vi "RDS Shore Remote.vi"() -> ()   [LabVIEW 2015]
uses:
  Libraries/3rd Party/NMEA_GPS/NMEA_GPRMC-data.ctl
  Libraries/3rd Party/NMEA_GPS/NMEA_LatitudeDirection.ctl
  Libraries/3rd Party/NMEA_GPS/NMEA_LongitudeDirection.ctl
  Libraries/RDS Instruments/Compass/Compass Data.ctl
  Libraries/RDS Child Messages/MCB/MCB Motor Status.ctl
  Libraries/RDS Child Messages/Mission Messages/Mission Controller State Control.ctl
  RDS Mission Controller Actor/Mission Controller Navigation State.ctl
  RDS Mission Controller Actor/MissionOp.ctl
  Libraries/RDS Child Messages/Helm/Helm Status Message/Helm Status Control.ctl
  Actors/RDS Helm Actor/RDS Helm Actor/Helm State.ctl
  Libraries/RDS Child Messages/Helm/Heading Command/Heading Command Cntrl.ctl
  Libraries/RDS Child Messages/Helm/Steering Command/Steering Command Cntrl.ctl
  Libraries/RDS Child Messages/PID Gains/PID Gains Control.ctl
  Libraries/RDS Instruments/AIP/AIP Status.ctl
  Libraries/RDS Instruments/AIP/AIP States.ctl
  Libraries/RDS Instruments/Battery/Battery Data.ctl
  Libraries/RDS Child Messages/Battery Data/Battery Status.ctl
  Actors/RDS Controller Actor/RDS Controller Actor/Controller.ctl
  SR_Overview.ctl
  SR_Thermal.ctl
  RDS Mission Controller Actor/Mission Controller Settings.ctl
  Libraries/GUI/Throttles.ctl
  RDS State Tracker/RDS State/RDS State.lvclass
  Libraries/RDS Framework/RDS Message Class/RDS Message.lvclass
  Libraries/RDS Serial Handler/RDS Serial Instrument.lvclass
  RDS Q Message.ctl
  SR-J-State.ctl
  Libraries/RDS Serial Handler/RDS Serial Frame.lvclass/RDS Serial Frame.ctl
  Libraries/RDS Serial Handler/RDS Serial Instrument.lvclass/RDS Serial Instrument.ctl
  RDS State Tracker/RDS State/RDS State.lvclass/RDS State.ctl
  Libraries/RDS Framework/RDS Message Class/RDS Message.lvclass/RDS Message.ctl
  Libraries/RDS Child Messages/Controller Message/Controller Message.lvclass
  Libraries/RDS Child Messages/Controller Message/Controller Message.lvclass/Controller Message.ctl
  Libraries/RDS Child Messages/State Sample Message/State Sample Message.lvclass
  Libraries/RDS Child Messages/State Sample Message/State Sample Message.lvclass/State Sample Message.ctl
  Libraries/RDS Framework/RDS Message ID.ctl
  Libraries/RDS Child Messages/PID Gains/PID Gains Set Message.lvclass
  Libraries/RDS Child Messages/PID Gains/PID Gains Set Message.lvclass/PID Gains Set Message.ctl
  Libraries/RDS Child Messages/Helm/Steering Command/Steering Command.lvclass
  Libraries/RDS Child Messages/Helm/Steering Command/Steering Command.lvclass/Steering Command.ctl
  Libraries/RDS Child Messages/Controller Message/Controller Message Type.ctl
  Libraries/RDS Child Messages/AIP Set Min Depth Message/AIP Set Min Depth Message.lvclass
  Libraries/RDS Child Messages/AIP Set Min Depth Message/AIP Set Min Depth Message.lvclass/AIP Set Min Depth Message.ctl
  Libraries/RDS Child Messages/Helm/Helm Limiter Message/Helm Limiter Msg.lvclass
  Libraries/RDS Child Messages/Helm/Helm Limiter Message/Helm Limiter Msg.lvclass/Helm Limiter Msg.ctl
  Libraries/RDS Framework/RDS Message Class/AIP Command.lvclass
  Libraries/RDS Framework/RDS Message Class/AIP Command Control.ctl
  Libraries/RDS Framework/RDS Message Class/AIP Command.lvclass/AIP Command.ctl
  <vilib>/Utility/inputDevices.llb/closeJoystick.vi
  Libraries/RDS Serial Handler/RDS Serial Frame.lvclass
  LSR Instrument Actor/LSR Instrument/LSR Instrument.lvlib
  LSR Transmission/LSR Transmission.lvlib
  Shore Library.lvlib
  Libraries/RDS Child Messages/RDS Child Messages.lvlib
  Compass Instrument/Compass Instrument.lvlib
  RDS Mission Controller Actor/RDS Mission Controller Actor.lvlib
  Actors/RDS Controller Actor/RDS Controller Actor/RDS Controller Actor.lvlib
  Libraries/RDS Instruments/RDS Instrument Library.lvlib
  Actors/RDS Helm Actor/RDS Helm Actor.lvlib
  Libraries/3rd Party/NMEA_GPS/NMEA.lvlib
  Libraries/RDS Child Messages/Mission Messages/Mission Controller State Message.lvclass
  Libraries/Geo/RDS Libraries.lvlib
panel:
  in  "Track":cluster{"Long":dbl[], "Lat":dbl[]}
  in  "btn_mission_maker":bool
  out "Joystick Connected":bool
  out "iHasControl":bool
  out "AIP controls":T1
  out "Seconds Ago":dbl format="%#.0g"
  out "Last Status Message":timestamp
  out "RoboDolf State":T2
  in  "Connect Joystick":bool
  out "LSR Connected":bool
  in  "Digi Connect":bool
  in  "Digi Serial Port":refnum<visa-resource-name>="COM11"
  in  "Tab Control":T3(tab)
  out "Overview":T4 {"Distance to Target" format="%.01f [meters]"; "Longitude" format="%.6g"; "Latitude" format="%.6g"; "Water Temp" format="%.0f [celcius]"; "Pitch" scale=45.0..-45.0; "Roll" scale=-20.0..20.0; "Current" format="%02.2f [amps]"; "Voltage" format="%02.2f [volts]"; "Capacity" format="%_1f [Percent]"; "Water Depth" format="%.01f [meters]"; "GPS Speed" format="%.01f [knots]"; "Compass" scale=0.36..360.0}
  out "Tx packet  length":i32(graph)
  out "Compass Data":T5
  out "GPRMC-data":T6={"TimeStamp"=timestamp(0 s since 1904-01-01), "Validity"=FALSE, "Latitude"=0.0, "Latitude-Direction"=enum."North", "Longitude"=0.0, "Longitude-Direction"=enum."East", "Speed in knots"=0.0, "True course"=0.0, "Date Stamp"=timestamp(0 s since 1904-01-01), "Magnetic Variation (East/West)"=0.0, "GPS Latitude"=0.0, "GPS Longitude"=0.0} {"GPS Longitude" format="%.6f"; "GPS Latitude" format="%.6f"; "Magnetic Variation (East/West)" format="%.02f [deg]"; "Date Stamp" format="%<%x>T"; "True course" format="%.02f [deg]"; "Speed in knots" format="%.02f [kts]"; "Longitude" format="%0.4f [long]"; "Latitude" format="%.04f [lat]"; "TimeStamp" format="%<%.2X>T"}
  in  "Compass Mag Dev":dbl
  in  "btn_set_mag_dev":bool
  in  "AIP Stop":bool
  in  "AIP Stow":bool
  in  "AIP Deploy":bool
  out "AS":bool
  out "FS":bool
  out "AP":bool
  out "FP":bool
  out "AIP Status":T9
  in  "AIP JD FP":bool
  in  "AIP JS FP":bool
  in  "AIP JS FS":bool
  in  "AIP JD FS":bool
  in  "AIP JD AP":bool
  in  "AIP JD AS":bool
  in  "AIP JS AS":bool
  in  "AIP JS AP":bool
  in  "AIP D FP":bool
  in  "AIP D FP 4":bool
  in  "AIP D AP":bool
  in  "AIP D FS":bool
  in  "AIP S AS":bool
  in  "AIP S AP":bool
  in  "AIP S FP":bool
  in  "AIP S FS":bool
  in  "AIP Min Depth":dbl
  in  "btn_set_aip_min_depth":bool
  out "Throttles":T11 {"STBD" scale=-1000.0..1000.0; "Port" scale=-1000.0..1000.0}
  out "Rudder Chart":sgl(graph)
  out "Hdng Chart":cluster{"Heading":sgl, "Current Heading":dbl}(graph) caption="Desired and Actual Heading Chart"
  out "Helm Status":T12 {"Gains"."D (Td)" format="%#_9f"; "Gains"."I (Ti)" format="%#_9f"; "Gains"."P (Kc)" format="%#.9f"}
  in  "btn_limiter_set":bool
  in  "Limter":dbl(slide) min=0.0 max=100.0 scale=0.0..100.0
  in  "Gains":T16 {"D (Td)" format="%#_9f"; "I (Ti)" format="%#_9f"; "P (Kc)" format="%#.9f"}
  in  "btn_gains set":bool
  in  "Steering Command":T15
  in  "btn_Send-Steer":bool
  in  "btn_show_annotes":bool caption="Show Annotes"
  in  "btn_show_loaded":bool caption="Show Loaded"
  in  "btn_upload_mission":bool
  in  "btn_show_buffer_1":bool caption="Show"
  in  "btn_load_buff_mission":bool
  out "XY Graph":cluster{dbl[], dbl[]}[](graph)
  out "Mission Controller State":T17 {"Mission"."GPS Longitude" format="%.6g"; "Mission"."GPS Latitude" format="%.6g"}
  in  "btn_mission_ReqControl":bool
  in  "btn_send settings":bool
  in  "Mission Controller Settings":T20
  in  "btn_mission_Relinquish":bool
  in  "btn_set_op_run":bool
  in  "MissionOp Index":i32
  in  "btn_Turneffe":bool
  in  "btn_beach1":bool
  in  "btn_beach 2":bool
  in  "btn_save_track":bool
  out "Mission Buffer":T19[](array[typedef]) {"GPS Longitude" format="%.6g"; "GPS Latitude" format="%.6g"}
  out "Voltage Chart":T21(graph)
  out "Pow Cap Chart":cluster{"Pack Current":sgl, "Pack Capacity":sgl}(graph) caption="Power and Capacity Chart"
  out "Battery Pack Info":T22
  out "Port Motor Data":T24
  out "STBD Motor":T24
  out "Thermal":T25
  out "Thermal WF":sgl[](graph)
  in  "btn-emergency-shutdown":bool
  in  "Shutdown Safety":bool
  in  "stop":bool
  # "SAMMUT TECHNOLOGIES LLC"
  # "RoboDolf State"
  # "Batteries"
  # "Actual Heading"
  # "Desired Heading"
  # "Throttle"
  # "PORT"
  # "STBD"
  # "FWD"
  # "PORT"
  # "STBD"
  # "AFT"
  # "Throttle -1000 to 1000\nRudder -100 to 100"
  # "MISSION BUFFER"
  # "Average 3.2 V (working)  3.65V-3.8V (peak )  2.5 V ( cut-off low)"
  # "All units in Celcuis"
  # "PORT"
  # "FWD"
  # "AFT"
  # "STBD"
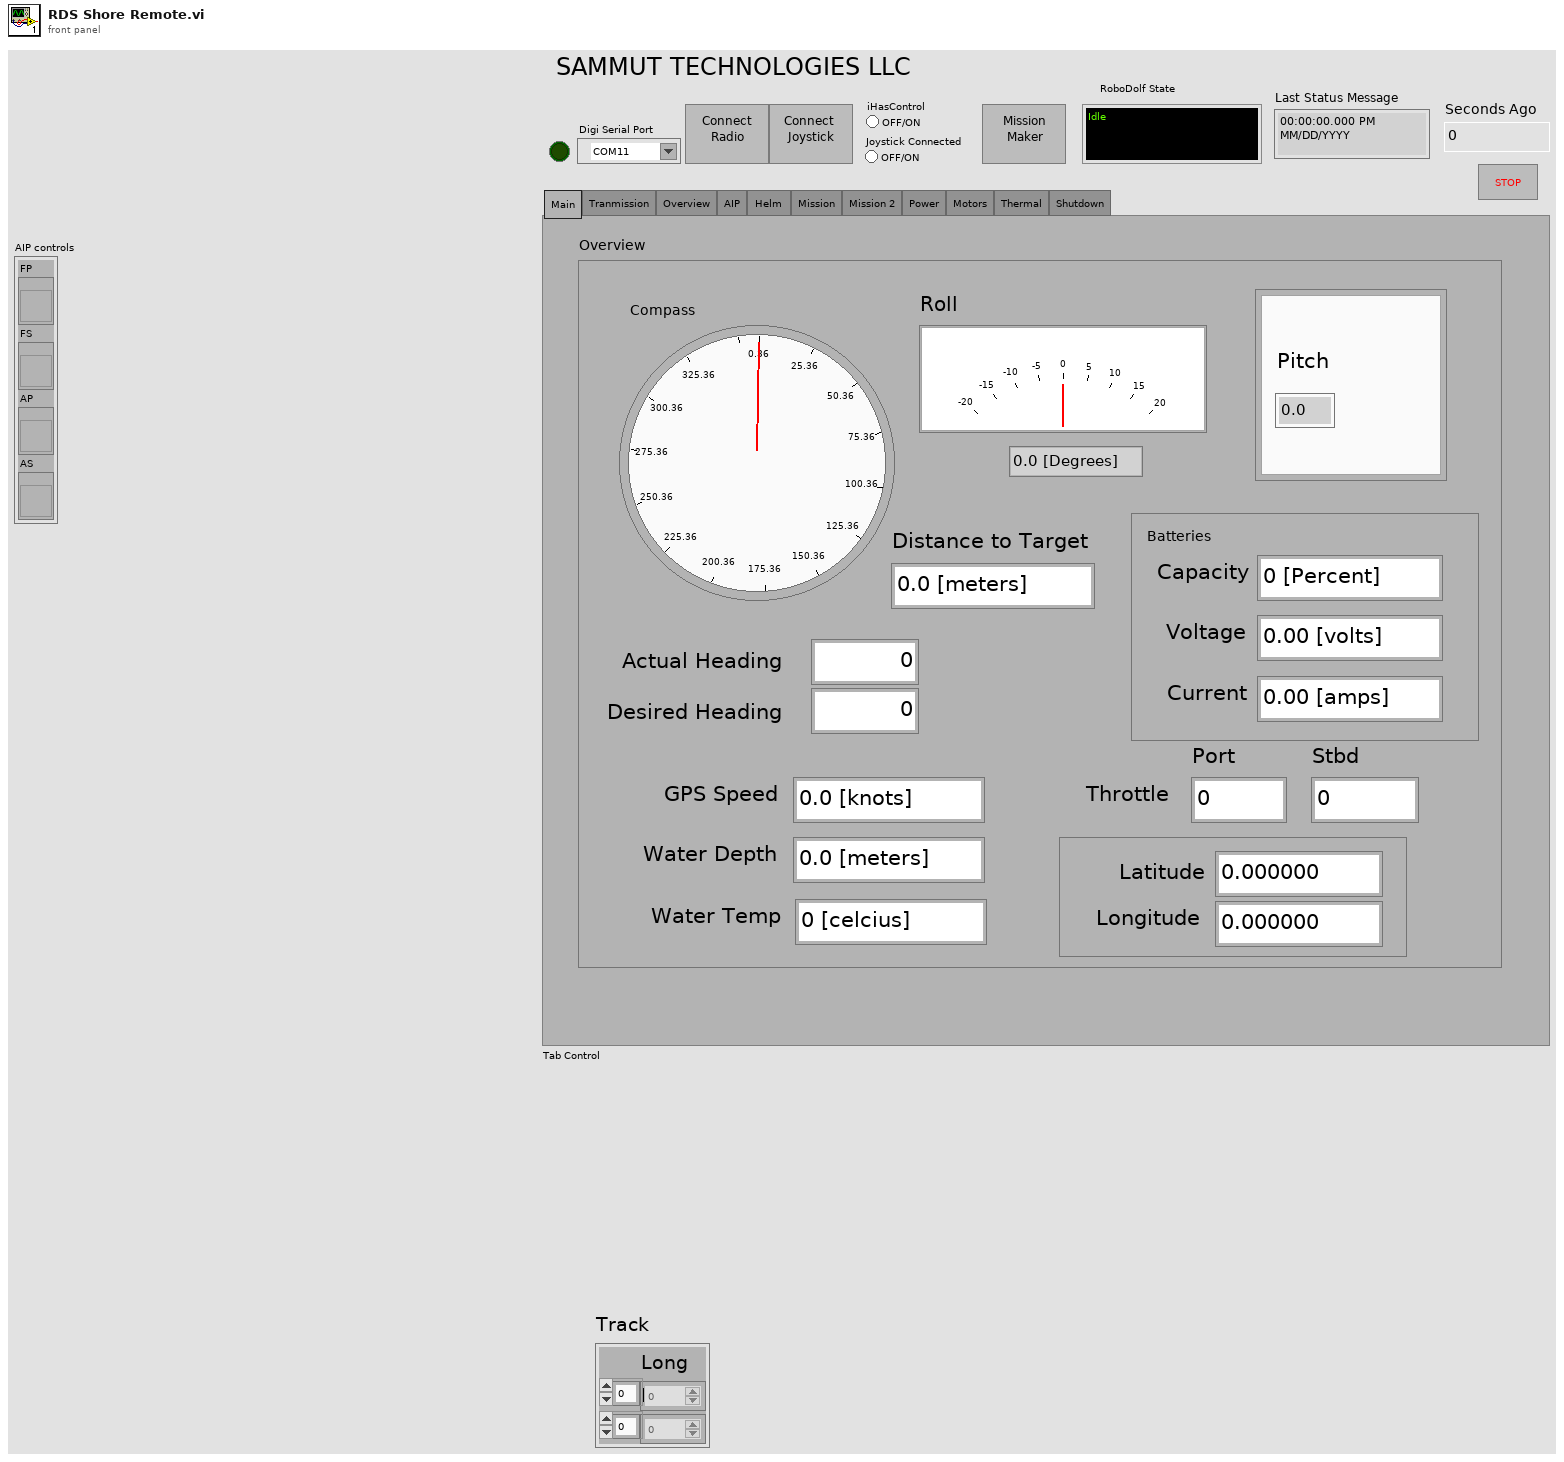
[diagram p1: front panel]
types:
  T1 = cluster{"FP":refnum<vi>, "FS":refnum<vi>, "AP":refnum<vi>, "AS":refnum<vi>}
  T2 = typedef "RDS Controller Actor.lvlib/Controller.ctl" = enum16{"Idle", "Local Remote Control", "Shore Remote Control", "Mission Control"}
  T3 = enum32{"Main", "Tranmission", "Overview", "AIP", "Helm ", "Mission", "Mission 2", "Power", "Motors", "Thermal", "Shutdown"}
  T4 = typedef "Shore Library.lvlib/SR_Overview.ctl" = cluster{"Throttle Stbd":dbl, "Compass":cluster{sgl, sgl}, "GPS Speed":dbl, "Water Depth":dbl, "Capacity":dbl, "Voltage":dbl, "Current":dbl, "Throttle Port":dbl, "Roll":sgl, "Pitch":sgl, "Water Temp":dbl, "Latitude":dbl, "Longitude":dbl, "Distance to Target":dbl}
  T5 = typedef "RDS Instrument Library.lvlib/Compass Data.ctl" = cluster{"Compass Heading":sgl, "pitch Angle":sgl, "roll Angle":sgl, "Temperature":sgl, "Depth":sgl, "Magnetic Field":sgl, "Magnetic Field X":sgl, "Magnetic Field Y":sgl, "Magnetic Field Z":sgl, "Acceleration":sgl, "Acceleration X":sgl, "Acceleration Y":sgl, "Gyro":sgl, "Gyro X":sgl, "Acceleration Z":sgl, "Gyro Y":sgl, "Raw Heading":sgl}
  T6 = typedef "RDS Libraries.lvlib/NMEA.lvlib/NMEA_GPRMC-data.ctl" = cluster{"TimeStamp":timestamp, "Validity":bool, "Latitude":dbl, "Latitude-Direction":T7, "Longitude":dbl, "Longitude-Direction":T8, "Speed in knots":sgl, "True course":sgl, "Date Stamp":timestamp, "Magnetic Variation (East/West)":sgl, "GPS Latitude":dbl, "GPS Longitude":dbl}
  T7 = typedef "RDS Libraries.lvlib/NMEA.lvlib/NMEA_LatitudeDirection.ctl" = enum16{"", "North", "South"}
  T8 = typedef "RDS Libraries.lvlib/NMEA.lvlib/NMEA_LongitudeDirection.ctl" = enum16{"", "East", "West"}
  T9 = typedef "RDS Instrument Library.lvlib/AIP Status.ctl" = cluster{"FWD Port":T10, "FWD Stbd":T10, "AFT Port":T10, "AFT Stbd":T10, "AIP Depth Min":u8}
  T10 = typedef "RDS Instrument Library.lvlib/AIP States.ctl" = enum16{"Deploy", "Deploying", "Deployed", "Stow", "Stowing", "Stowed", "Fault", "brakeOnStow", "breakOnDeploy", "Stopped", "Stopping"}
  T11 = typedef "RDS Libraries.lvlib/Throttles.ctl" = cluster{"Port":dbl, "STBD":dbl}
  T12 = typedef "RDS Child Messages.lvlib/Helm Status Control.ctl" = cluster{"Helm State":T13, "Heading Command Control":T14, "Steering Command Control":T15, "Last Command Time":timestamp, "Gains":T16, "Current Heading":dbl, "Port Throttle":i16, "STBD Throttle":i16, "Limiter":dbl}
  T13 = typedef "RDS Helm Actor.lvlib/Helm State.ctl" = enum16{"Idle", "Executing Heading Command", "Executing Steering Command"}
  T14 = typedef "RDS Child Messages.lvlib/Heading Command Cntrl.ctl" = cluster{"Throttle":i16, "Heading":sgl, "Duration (s)":i16}
  T15 = typedef "RDS Child Messages.lvlib/Steering Command Cntrl.ctl" = cluster{"Throttle":i16, "Rudder":i8, "Duration (s)":u16}
  T16 = typedef "RDS Child Messages.lvlib/PID Gains Control.ctl" = cluster{"P (Kc)":sgl, "I (Ti)":sgl, "D (Td)":sgl}
  T17 = typedef "RDS Child Messages.lvlib/Mission Controller State Message.lvclass/Mission Controller State Control.ctl" = cluster{"iHasControl":bool, "controlTimer":timestamp, "Nav State":T18, "Current MissionOp Index":i32, "Mission":T19[], "Distance to Target":dbl, "Seconds to Timeout":dbl}
  T18 = typedef "RDS Mission Controller Actor.lvlib/Mission Controller Navigation State.ctl" = cluster{"GPS Latitude":ext, "GPS Longitude":ext, "Compass Heading":dbl, "Speed":dbl}
  T19 = typedef "RDS Mission Controller Actor.lvlib/MissionOp.ctl" = cluster{"MissionOp Type":enum16{"Waypoint", "Loiter", "Wait", "Deploy AIP", "Stow AIP"}, "Duration (s)":u16, "Throttle":i16, "GPS Latitude":dbl, "GPS Longitude":dbl, "Loiter Range (m)":u16}
  T20 = typedef "RDS Mission Controller Actor.lvlib/Mission Controller Settings.ctl" = cluster{"Waypoint Radius (m)":dbl}
  T21 = cluster{"Max Cell Voltage":sgl, "Min Cell Voltage":sgl}
  T22 = typedef "RDS Instrument Library.lvlib/Battery Data.ctl" = cluster{"Battery Status":T23, "Pack Voltage":sgl, "Pack Current":sgl, "Pack Capacity":sgl, "Max Cell Temp":sgl, "Min Cell Temp":sgl, "Max Cell Voltage":sgl, "Min Cell Voltage":sgl}
  T23 = typedef "RDS Instrument Library.lvlib/Battery Status.ctl" = enum16{"Pack Normal", "Alarm: Cell temp too high", "Alarm: Pack voltage too high", "Warn: Pack voltage too high ", "Alarm: Pack voltage too low", "Warn: Pack voltage low", "Alarm Pack current too high", "Warn: Pack current too high ", "Fault: Pack to chassis connection detected", "Fault: Pack to cell connection error", "Fautl: System error"}
  T24 = typedef "RDS Child Messages.lvlib/MCB Motor Status.ctl" = cluster{"Motor Power":i16, "Motor Command":i16, "Battery Volts":sgl, "Battery Amps":sgl, "Motor Amps":sgl, "MCU Temp":i16, "Heatsink Temp":i16, "Fault Flags":u16, "StatusFlags":u16}
  T25 = typedef "Shore Library.lvlib/SR_Thermal.ctl" = cluster{"Port MC":sgl, "Stbd MC":sgl, "Batt":sgl, "MFB":sgl}
  T26 = enum8{"Enabled", "Disabled", "Disabled and Grayed Out"}
  T27 = typedef "Shore Library.lvlib/SR-J-State.ctl" = cluster{"iHasControl":bool, "cntrlReq":bool, "JS Cur State":cluster{"axis info":cluster{"X axis":i32, "Y axis":i32, "Z axis":i32, "X axis rotation":i32, "Y axis rotation":i32, "Z axis rotation":i32, "U axis":i32, "V axis":i32}, "button info":cluster{"button 1":bool, "button 2":bool, "button 3":bool, "button 4":bool, "button 5":bool, "button 6":bool, "button 7":bool, "button 8":bool, "button 9":bool, "button 10":bool, "button 11":bool, "button 12":bool, "button 13":bool, "button 14":bool, "button 15":bool, "button 16":bool, "button 17":bool, "button 18":bool, "button 19":bool, "button 20":bool, "button 21":bool, "button 22":bool, "button 23":bool, "button 24":bool, "button 25":bool, "button 26":bool, "button 27":bool, "button 28":bool, "button 29":bool, "button 30":bool, "button 31":bool, "button 32":bool}, "direction info":cluster{"pov 1":i32, "pov 2":i32, "pov 3":i32, "pov 4":i32}}, "JS Prev State":cluster{"axis info":cluster{"X axis":i32, "Y axis":i32, "Z axis":i32, "X axis rotation":i32, "Y axis rotation":i32, "Z axis rotation":i32, "U axis":i32, "V axis":i32}, "button info":cluster{"button 1":bool, "button 2":bool, "button 3":bool, "button 4":bool, "button 5":bool, "button 6":bool, "button 7":bool, "button 8":bool, "button 9":bool, "button 10":bool, "button 11":bool, "button 12":bool, "button 13":bool, "button 14":bool, "button 15":bool, "button 16":bool, "button 17":bool, "button 18":bool, "button 19":bool, "button 20":bool, "button 21":bool, "button 22":bool, "button 23":bool, "button 24":bool, "button 25":bool, "button 26":bool, "button 27":bool, "button 28":bool, "button 29":bool, "button 30":bool, "button 31":bool, "button 32":bool}, "direction info":cluster{"pov 1":i32, "pov 2":i32, "pov 3":i32, "pov 4":i32}}, "device ID":refnum<k1>, "controlTimer":timestamp, "halfSecTimer":timestamp, "AIPcmdTimer":timestamp, "Joystick Connected":bool}
  T28 = cluster{"axis info":cluster{"X axis":i32, "Y axis":i32, "Z axis":i32, "X axis rotation":i32, "Y axis rotation":i32, "Z axis rotation":i32, "U axis":i32, "V axis":i32}, "button info":cluster{"button 1":bool, "button 2":bool, "button 3":bool, "button 4":bool, "button 5":bool, "button 6":bool, "button 7":bool, "button 8":bool, "button 9":bool, "button 10":bool, "button 11":bool, "button 12":bool, "button 13":bool, "button 14":bool, "button 15":bool, "button 16":bool, "button 17":bool, "button 18":bool, "button 19":bool, "button 20":bool, "button 21":bool, "button 22":bool, "button 23":bool, "button 24":bool, "button 25":bool, "button 26":bool, "button 27":bool, "button 28":bool, "button 29":bool, "button 30":bool, "button 31":bool, "button 32":bool}, "direction info":cluster{"pov 1":i32, "pov 2":i32, "pov 3":i32, "pov 4":i32}}
  T29 = typedef "RDS Q Message.ctl" = enum16{"RDS Message", "Shutdown"}
  T30 = cluster{"Msg Type":T29, "RDS Msg":refnum<class "RDS Message.lvclass">}
  T31 = cluster{"Name":string, "Color":u32, "Style":u8, "Point Style":u8, "Name Visible":bool, "Allow Drag":bool, "Annotation Mode":u32, "Plot":i32, "Index":i32, "Position":cluster{"X":dbl, "Y":dbl}, "X Scale":u32, "Y Scale":u32, "Show Arrow":bool, "Lock Name":bool, "Plot Area":i32, "Label Offset":cluster{"X":dbl, "Y":dbl}}[]
  T32 = enum32{"Invalid", "Standard", "Closed", "Hidden", "Minimized", "Maximized"}
  T33 = typedef "RDS Child Messages.lvlib/RDS Message ID.ctl" = enum16{"RDS Hello World", "String Message", "AIP_Status", "AIP_Command", "GPS_Data", "MCB_Command", "MCB_Status", "Compass_Data", "Depth_Data", "Battery_Data", "Contoller_State", "Set_Mag_Dev", "BTB_Shutdown", "State_Sample_Request", "State_Sample", "PID_Gains_Set", "Helm_Limiter_Set", "Helm_Heading_Command", "Helm_Steering_Command", "Helm_Status", "Controller_Message", "AIP_Set_Min_Depth", "Mission_Controller_State", "Mission_Upload", "Mission_Set_Op_and_Run", "Mission_Settings_Set"}
  T34 = typedef "RDS Child Messages.lvlib/Controller Message.lvclass/Controller Message Type.ctl" = enum16{"Control Relinquish Request", "Control Relinquish Command", "Control Request", "Control Granted"}
  T35 = typedef "RDS Child Messages.lvlib/AIP Command Control.ctl" = enum16{"Stow", "Deploy", "Stop", "Validate Sensors", "Jog Deploy FP", "Jog Stow FP", "Jog Deploy FS", "Jog Stow FS", "Jog Deploy AP", "Jog Stow AP", "Jog Deploy AS", "Jog Stow AS", "Deploy FP", "Deploy FS", "Deploy AP", "Deploy AS", "Stow FP", "Stow FS", "Stow AP", "Stow AS"}
  T36 = cluster{"RDS Shore Remote Msg":T29, "RDS Child Messages.lvlib:RDS Message.lvclass":refnum<class "RDS Message.lvclass">}
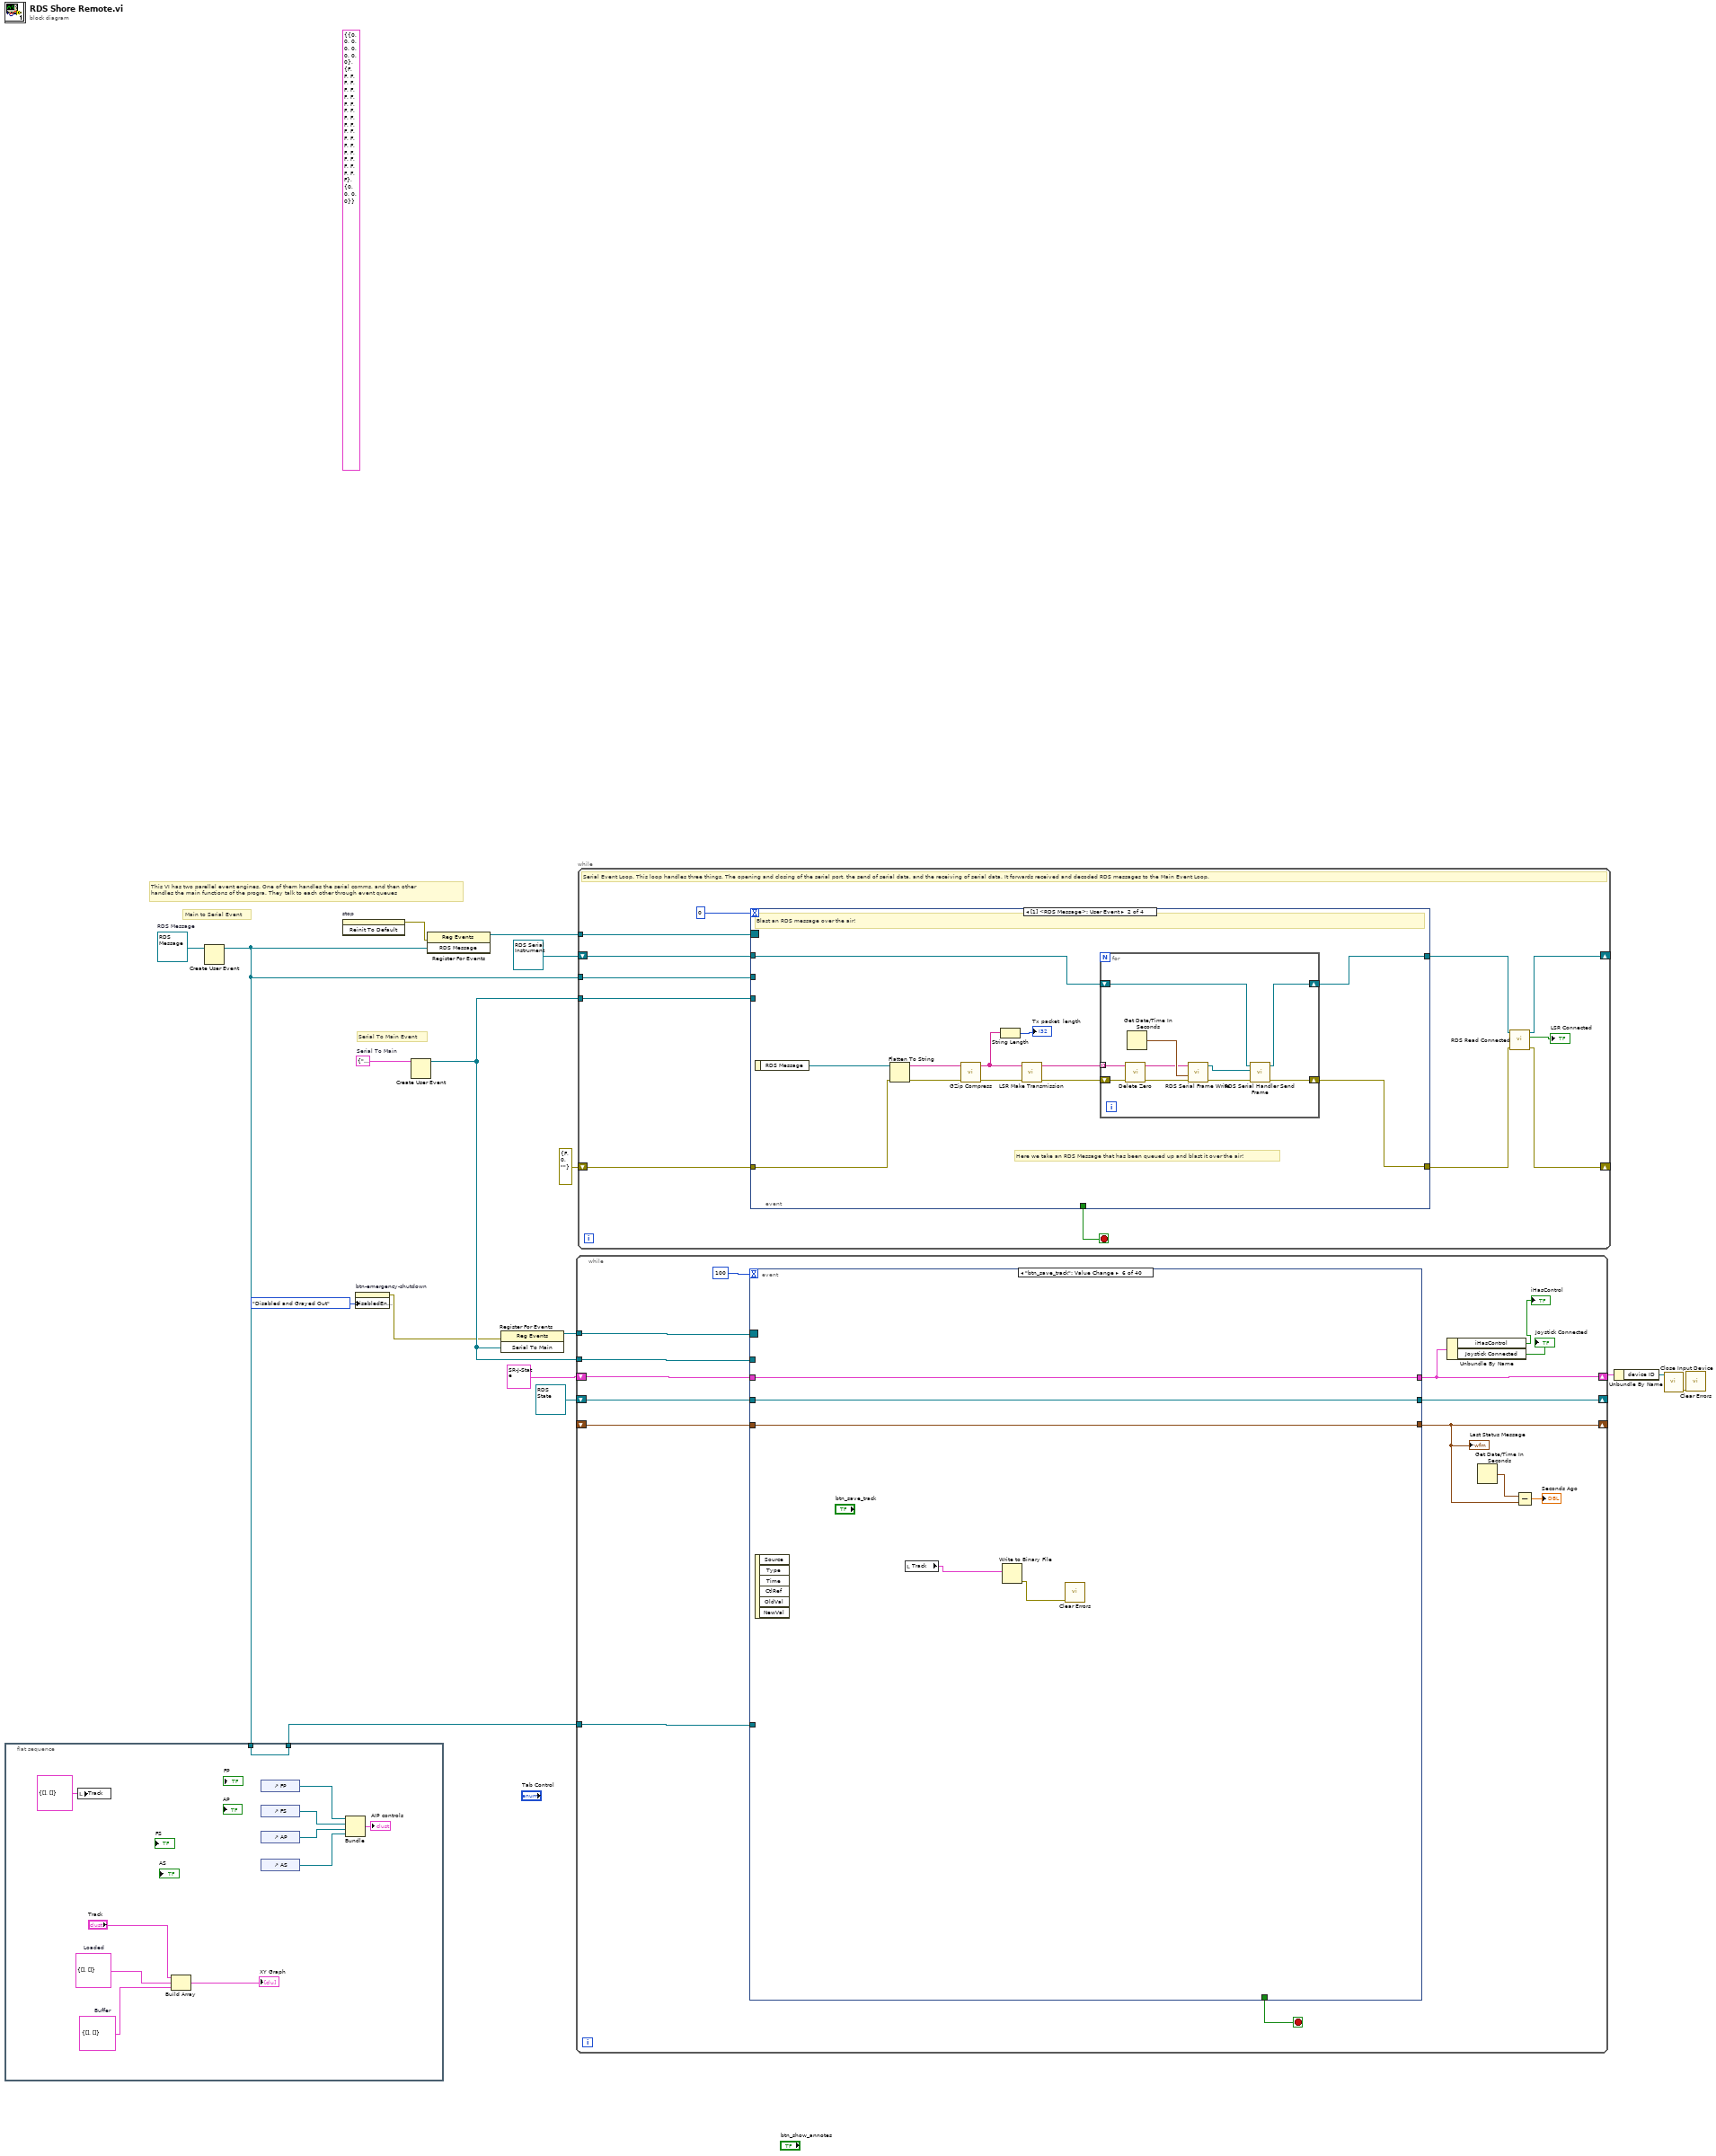
[diagram p0: block diagram]
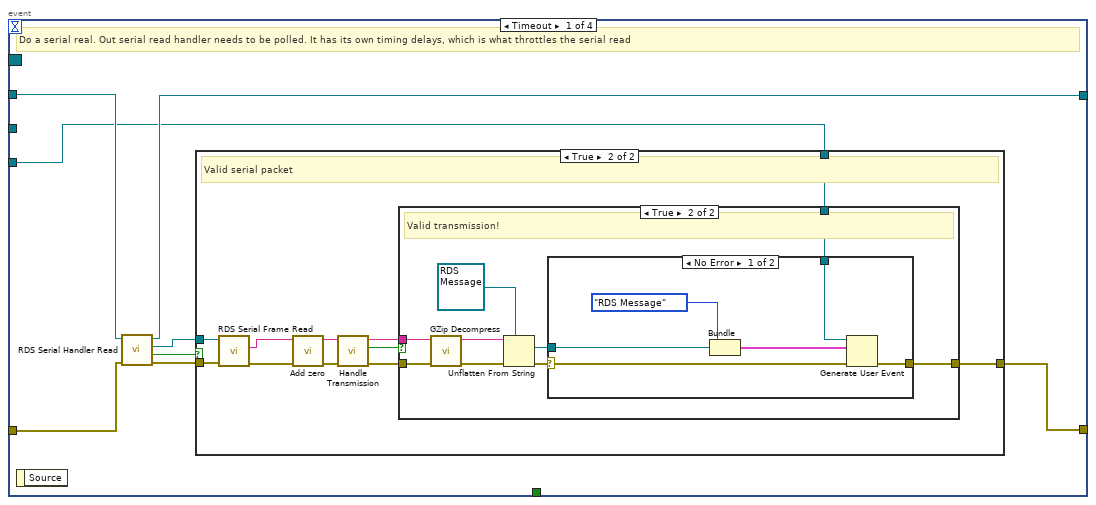
[diagram p2: hidden frame]
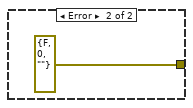
[diagram p5: hidden frame]
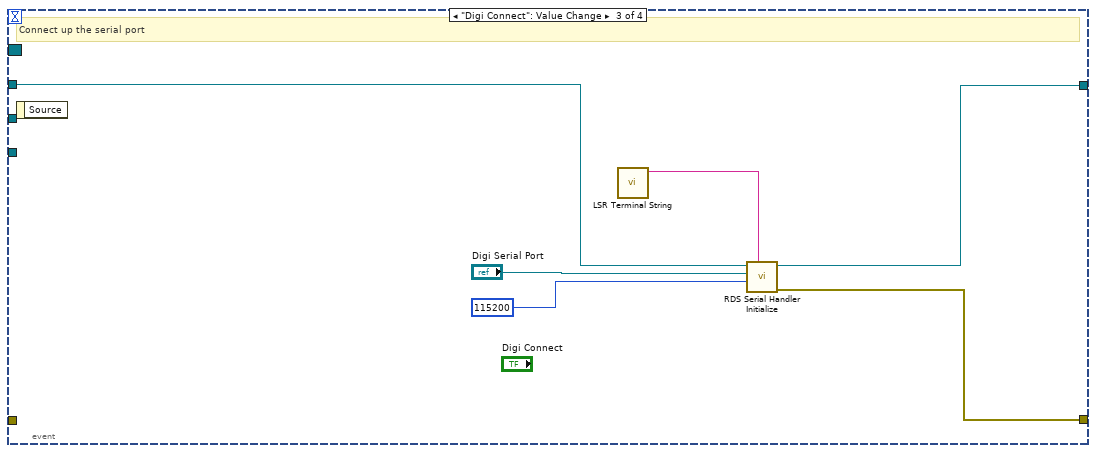
[diagram p6: hidden frame]
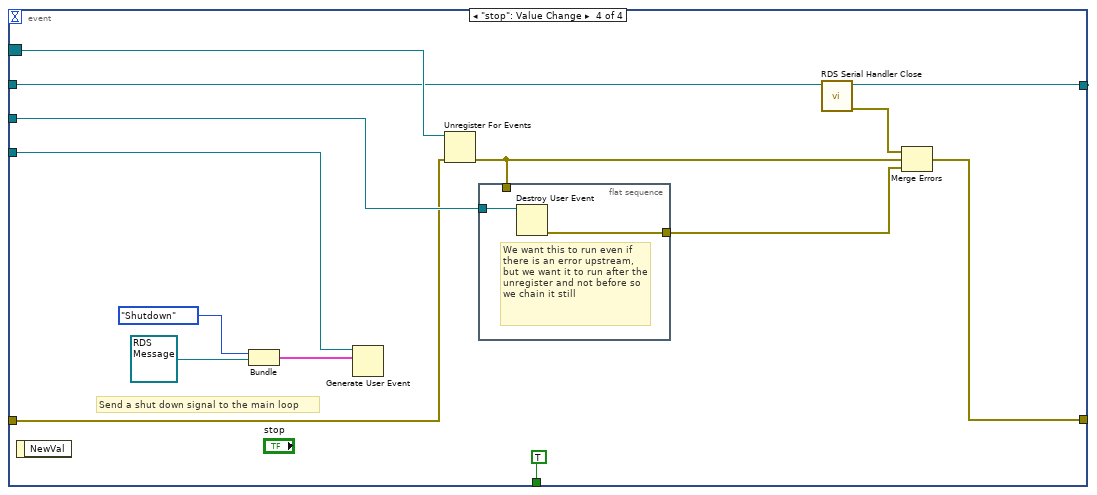
[diagram p7: hidden frame]
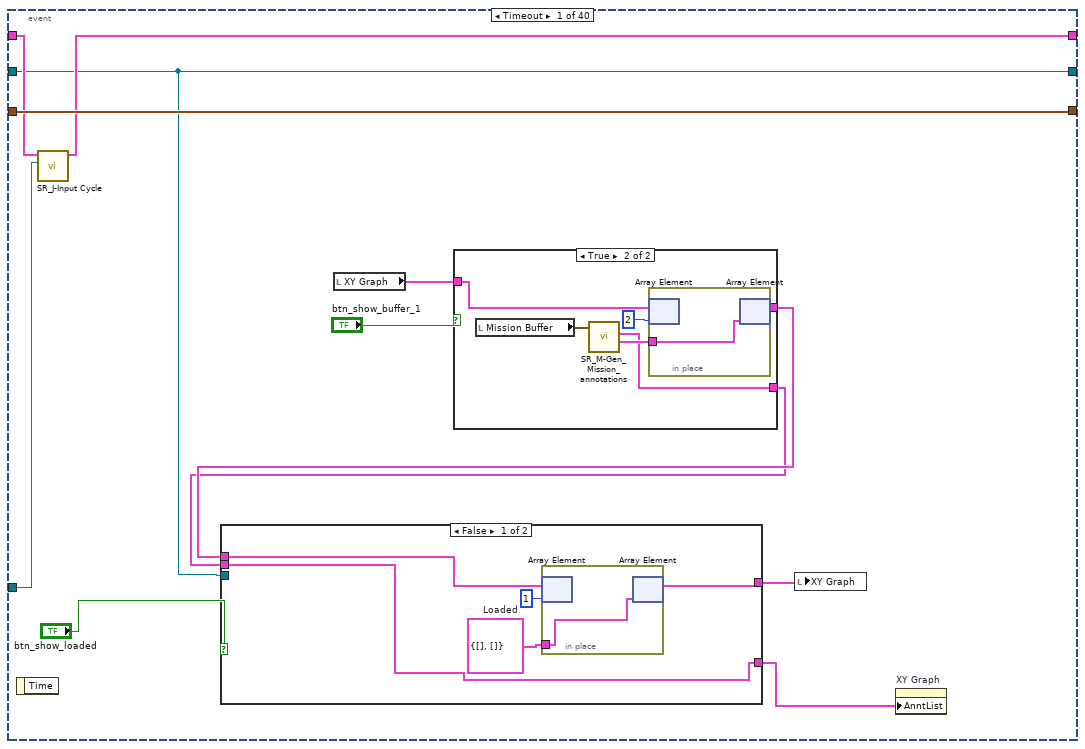
[diagram p8: hidden frame]
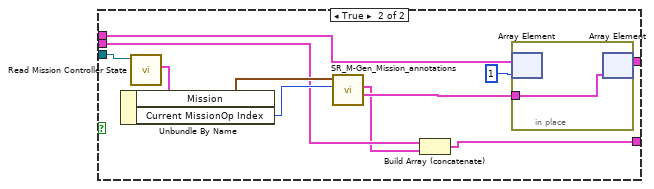
[diagram p9: hidden frame]
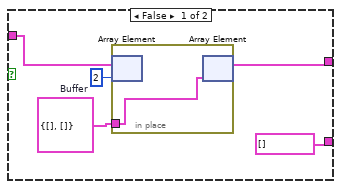
[diagram p10: hidden frame]
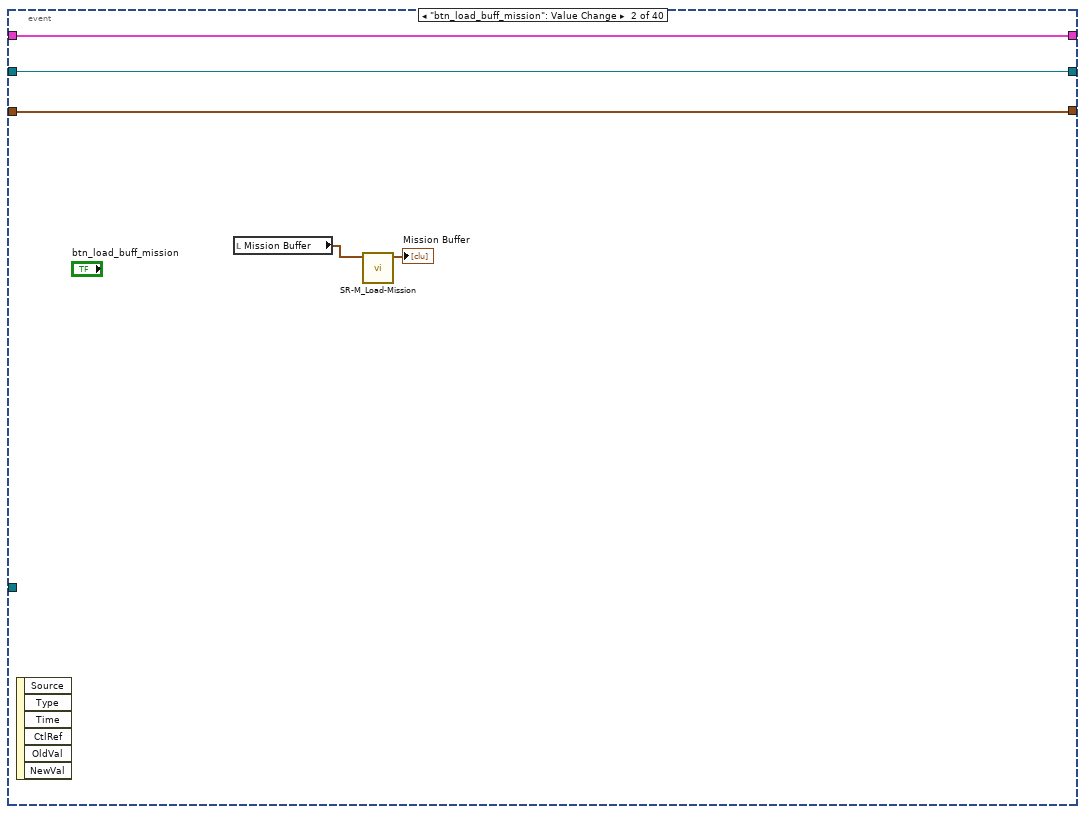
[diagram p11: hidden frame]
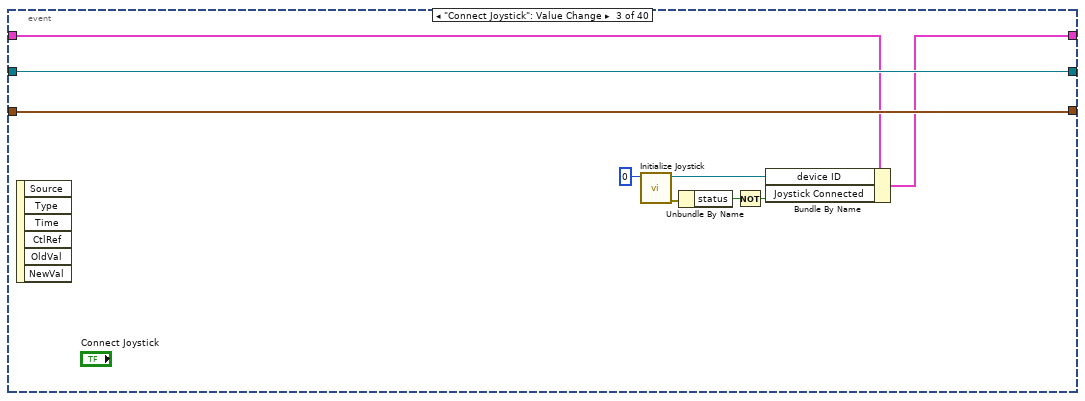
[diagram p12: hidden frame]
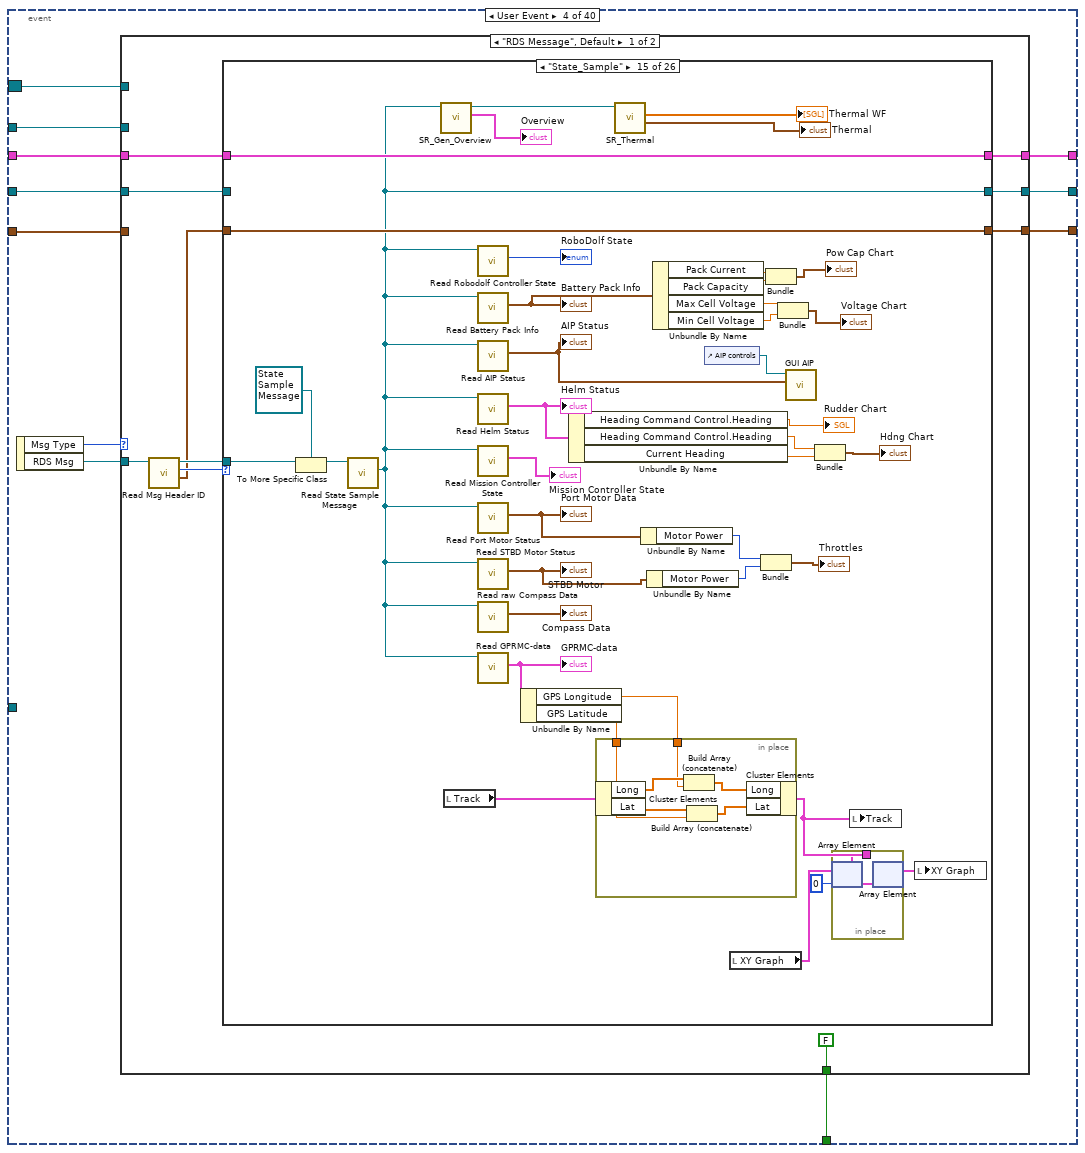
[diagram p13: hidden frame]
diagram:
  (unwired) T28 {"axis info"={"X axis"=0, "Y axis"=0, "Z axis"=0, "X axis rotation"=0, "Y axis rotation"=0, "Z axis rotation"=0, "U axis"=0, "V axis"=0}, "button info"={"button 1"=FALSE, "button 2"=FALSE, "button 3"=FALSE, "button 4"=FALSE, "button 5"=FALSE, "button 6"=FALSE, "button 7"=FALSE, "button 8"=FALSE, "button 9"=FALSE, "button 10"=FALSE, "button 11"=FALSE, "button 12"=FALSE, "button 13"=FALSE, "button 14"=FALSE, "button 15"=FALSE, "button 16"=FALSE, "button 17"=FALSE, "button 18"=FALSE, "button 19"=FALSE, "button 20"=FALSE, "button 21"=FALSE, "button 22"=FALSE, "button 23"=FALSE, "button 24"=FALSE, "button 25"=FALSE, "button 26"=FALSE, "button 27"=FALSE, "button 28"=FALSE, "button 29"=FALSE, "button 30"=FALSE, "button 31"=FALSE, "button 32"=FALSE}, "direction info"={"pov 1"=0, "pov 2"=0, "pov 3"=0, "pov 4"=0}} ("Joystick Prev State")
  w12 = T30 {"Msg Type"=enum."RDS Message", "RDS Msg"=refnum}  # Serial To Main
  w14 = refnum<class "RDS Message.lvclass"> refnum  # RDS Message
  # "Main to Serial Event"
  # "Serial To Main Event"
  # "This VI has two parellel event engines. One of them handles the serial comms, and then other \nhandles the main functions of the progra. They talk to each other through event queues"
  n1 = flat-sequence {
    tunnel: w9 -> [w23]
    tunnel: [w23] -> w8
    frame #0 {
      w20 = cluster{dbl[], dbl[]} {[], []}  # Buffer
      w19 = cluster{dbl[], dbl[]} {[], []}  # Loaded
      n2 = local write "Track"(cluster{dbl[], dbl[]} {[], []} ("Track")) -> ()
      n3 = Build Array("Track", w19, w20) -> (→"XY Graph":cluster{"Long":dbl[], "Lat":dbl[]}[])
      n4 = control-ref of="FP"() -> (w24:refnum<vi>)
      n5 = control-ref of="FS"() -> (w25:refnum<vi>)
      n6 = control-ref of="AP"() -> (w26:refnum<vi>)
      n7 = control-ref of="AS"() -> (w27:refnum<vi>)
      n8 = Bundle("FP"=w24, "FS"=w25, "AP"=w26, "AS"=w27) -> (→"AIP controls":T1)  [unwired: 1 in]
    }
  }
  n9 = Create User Event(user event datatype=w14) -> (user event=w9:refnum<user-event>)  [unwired: 1 in, 1 out]
  n10 = invoke on="stop" class="Bool" method="Reinit To Default"() -> (error out=w11:errorcluster)  [unwired: 3 in, 2 out]
  n11 = property on="btn-emergency-shutdown" class="Bool"("DisabledEnum"=T26."Disabled and Grayed Out" ("Disabled")) -> (error out=w1:errorcluster)  [unwired: 2 in, 1 out]
  n12 = Create User Event(user event datatype=w12) -> (user event=w10:refnum<user-event>)  [unwired: 1 in, 1 out]
  n13 = register-events(error in=w11, w9) -> (reference out=w15:refnum<event-registration>)  [unwired: 1 in, 1 out]
  n14 = register-events(error in=w1, w10) -> (reference out=w16:refnum<event-registration>)  [unwired: 1 in, 1 out]
  n15 = while {
    shift-right: [w37] -> _
    shift-left: refnum<class "RDS State.lvclass"> refnum ("RDS Child Messages.lvlib:RDS State.lvclass") -> [w42]
    shift-right: [w31] -> w5
    shift-left: T27 {"iHasControl"=FALSE, "cntrlReq"=FALSE, "JS Cur State"={"axis info"={"X axis"=0, "Y axis"=0, "Z axis"=0, "X axis rotation"=0, "Y axis rotation"=0, "Z axis rotation"=0, "U axis"=0, "V axis"=0}, "button info"={"button 1"=FALSE, "button 2"=FALSE, "button 3"=FALSE, "button 4"=FALSE, "button 5"=FALSE, "button 6"=FALSE, "button 7"=FALSE, "button 8"=FALSE, "button 9"=FALSE, "button 10"=FALSE, "button 11"=FALSE, "button 12"=FALSE, "button 13"=FALSE, "button 14"=FALSE, "button 15"=FALSE, "button 16"=FALSE, "button 17"=FALSE, "button 18"=FALSE, "button 19"=FALSE, "button 20"=FALSE, "button 21"=FALSE, "button 22"=FALSE, "button 23"=FALSE, "button 24"=FALSE, "button 25"=FALSE, "button 26"=FALSE, "button 27"=FALSE, "button 28"=FALSE, "button 29"=FALSE, "button 30"=FALSE, "button 31"=FALSE, "button 32"=FALSE}, "direction info"={"pov 1"=0, "pov 2"=0, "pov 3"=0, "pov 4"=0}}, "JS Prev State"={"axis info"={"X axis"=0, "Y axis"=0, "Z axis"=0, "X axis rotation"=0, "Y axis rotation"=0, "Z axis rotation"=0, "U axis"=0, "V axis"=0}, "button info"={"button 1"=FALSE, "button 2"=FALSE, "button 3"=FALSE, "button 4"=FALSE, "button 5"=FALSE, "button 6"=FALSE, "button 7"=FALSE, "button 8"=FALSE, "button 9"=FALSE, "button 10"=FALSE, "button 11"=FALSE, "button 12"=FALSE, "button 13"=FALSE, "button 14"=FALSE, "button 15"=FALSE, "button 16"=FALSE, "button 17"=FALSE, "button 18"=FALSE, "button 19"=FALSE, "button 20"=FALSE, "button 21"=FALSE, "button 22"=FALSE, "button 23"=FALSE, "button 24"=FALSE, "button 25"=FALSE, "button 26"=FALSE, "button 27"=FALSE, "button 28"=FALSE, "button 29"=FALSE, "button 30"=FALSE, "button 31"=FALSE, "button 32"=FALSE}, "direction info"={"pov 1"=0, "pov 2"=0, "pov 3"=0, "pov 4"=0}}, "device ID"=refnum, "controlTimer"=timestamp(0 s since 1904-01-01), "halfSecTimer"=timestamp(0 s since 1904-01-01), "AIPcmdTimer"=timestamp(0 s since 1904-01-01), "Joystick Connected"=FALSE} ("Cluster") -> [w41]
    tunnel: w16 -> [w40]
    tunnel: w8 -> [w38]
    tunnel: w10 -> [w36]
    shift-right: [w34] -> _
    shift-left: _ -> [w35]
    stop <- w39 stop-if-true
    n16 = event shown="[5] \"btn_save_track\": Value Change" {
      selector: w40 -> [_ _ _ w110 _ _ _ _ _ _ _ _ _ _ _ _ _ _ _ _ _ _ _ _ _ _ _ _ _ _ _ _ _ _ _ _ _ _ _ _]
      dyn-events: _ -> [_ _ _ _ _ _ _ _ _ _ _ _ _ _ _ _ _ _ _ _ _ _ _ _ _ _ _ _ _ _ _ _ _ _ _ _ _ _ _ _]
      timeout: 100 -> [_ _ _ _ _ _ _ _ _ _ _ _ _ _ _ _ _ _ _ _ _ _ _ _ _ _ _ _ _ _ _ _ _ _ _ _ _ _ _ _]
      tunnel: w42 -> [w45 w90 w99 w106 w273 w281 w299 w303 w311 w322 w329 w336 w343 w354 w360 w371 w386 w401 w407 w418 w429 w441 w452 w463 w474 w485 w496 w507 w518 w529 w540 w551 w562 w573 w584 w595 w606 w617 w628 w639]
      tunnel: [w52 w91 w95 w108 w274 w282 w300 w304 w312 w323 w330 w337 w344 w355 w361 w372 w387 w402 w408 w419 w430 w431 w442 w453 w464 w475 w486 w497 w508 w519 w530 w541 w552 w563 w574 w585 w596 w607 w618 w629] -> w31
      tunnel: w41 -> [w53 w91 w97 w111 w274 w282 w300 w304 w312 w323 w330 w337 w344 w355 w361 w372 w387 w402 w408 w419 w430 w431 w442 w453 w464 w475 w486 w497 w508 w519 w530 w541 w552 w563 w574 w585 w596 w607 w618 w629]
      tunnel: [_ _ _ w109 _ _ _ _ _ _ _ _ _ _ _ _ _ _ _ _ _ _ _ _ _ _ _ _ _ _ _ _ _ _ _ _ _ _ _ _] -> w39
      tunnel: w38 -> [w54 _ _ _ w269 _ _ _ w307 w318 _ _ _ w346 w357 w369 w374 w388 w404 w409 w421 w433 w444 w455 w466 w477 w488 w499 w510 w521 w532 w543 w554 w565 w576 w587 w598 w609 w620 w631]
      tunnel: [w45 w90 w99 w107 w273 w281 w299 w303 w311 w322 w329 w336 w343 w354 w360 w371 w386 w401 w407 w418 w429 w441 w452 w463 w474 w485 w496 w507 w518 w529 w540 w551 w562 w573 w584 w595 w606 w617 w628 w639] -> w37
      tunnel: w36 -> [_ _ _ w104 _ _ _ _ _ _ _ _ _ _ _ _ _ _ _ _ _ _ _ _ _ _ _ _ _ _ _ _ _ _ _ _ _ _ _ _]
      tunnel: [w55 w89 w98 w102 w272 w280 w298 w302 w310 w321 w328 w335 w342 w353 w359 w370 w385 w400 w406 w417 w428 w440 w451 w462 w473 w484 w495 w506 w517 w528 w539 w550 w561 w572 w583 w594 w605 w616 w627 w638] -> w34
      tunnel: w35 -> [w55 w89 w98 w101 w272 w280 w298 w302 w310 w321 w328 w335 w342 w353 w359 w370 w385 w400 w406 w417 w428 w440 w451 w462 w473 w484 w495 w506 w517 w528 w539 w550 w561 w572 w583 w594 w605 w616 w627 w638]
      event Timeout {
        n17 = event-data() -> ()  [unwired: 1 in, 1 out]
        n18 = call "SR_J-Input Cycle.vi"("RDS Msg Q in"=w54, "Joystick"=w53) -> ("Joystick Out"=w52:T27)  [unwired: 7 in, 2 out]
        n19 = local read "XY Graph"() -> (w50:cluster{dbl[], dbl[]}[])
        n20 = case shown="True" "btn_show_buffer_1" {
          tunnel: w50 -> [w77 w85]
          tunnel: [T31 [] ("Mission Annotation") w81] -> w44
          tunnel: [w74 w80] -> w46
          frame False {
            w75 = cluster{dbl[], dbl[]} {[], []}  # Buffer
            n21 = in-place {
              in-place-border: w75 -> [w79]
              n22 = in-place-array #1(w77, 2) -> ()  [unwired: 1 out]
              n23 = in-place-array #1(w79) -> (w74:cluster{dbl[], dbl[]}[])  [unwired: 1 out]
            }
          }
          frame True {
            n24 = local read "Mission Buffer"() -> (w83:T19[])
            n25 = call "SR_M-Gen_Mission_annotations.vi"("Mission In"=w83) -> ("Mission Path"=w82:cluster{dbl[], dbl[]}, "Mission Annotation"=w81:T31)  [unwired: 8 in, 1 out]
            n26 = in-place {
              in-place-border: w82 -> [w86]
              n27 = in-place-array #2(w85, 2) -> ()  [unwired: 1 out]
              n28 = in-place-array #2(w86) -> (w80:cluster{dbl[], dbl[]}[])  [unwired: 1 out]
            }
          }
        }
        n29 = case shown="False" "btn_show_loaded" {
          tunnel: w46 -> [w60 w72]
          tunnel: [w56 w62] -> w48
          tunnel: [w57 w69] -> w49
          tunnel: w45 -> [_ w68]
          tunnel: w44 -> [w56 w64]
          frame False {
            w58 = cluster{dbl[], dbl[]} {[], []}  # Loaded
            n30 = in-place {
              in-place-border: w58 -> [w61]
              n31 = in-place-array #3(w60, 1) -> ()  [unwired: 1 out]
              n32 = in-place-array #3(w61) -> (w57:cluster{dbl[], dbl[]}[])  [unwired: 1 out]
            }
          }
          frame True {
            n33 = call "Read Mission Controller State.vi"("RDS State in"=w68) -> ("Mission Controller State"=w67:T17)  [unwired: 8 in, 2 out]
            n34 = Unbundle By Name(w67) -> ("Mission"=w66:T19[], "Current MissionOp Index"=w65:i32)
            n35 = call "SR_M-Gen_Mission_annotations.vi"("Op Index"=w65, "Mission In"=w66) -> ("Mission Path"=w70:cluster{dbl[], dbl[]}, "Mission Annotation"=w63:T31)  [unwired: 7 in, 1 out]
            n36 = Build Array (concatenate)(w64, w63) -> (w62:T31)
            n37 = in-place {
              in-place-border: w70 -> [w73]
              n38 = in-place-array #4(w72, 1) -> ()  [unwired: 1 out]
              n39 = in-place-array #4(w73) -> (w69:cluster{dbl[], dbl[]}[])  [unwired: 1 out]
            }
          }
        }
        n40 = local write "XY Graph"(w49) -> ()
        n41 = property on="XY Graph" class="XYGraph (strict)"("AnntList"=w48) -> ()  [unwired: 2 in, 2 out]
      }
      event "btn_load_buff_mission": Value Change {
        n42 = event-data() -> ()  [unwired: 1 in, 6 out]
        n43 = local read "Mission Buffer"() -> (w87:T19[])
        n44 = call "SR-M_Load-Mission.vi"("Mission In in"=w87) -> ("Mission In out"=→"Mission Buffer":T19[])  [unwired: 10 in]
      }
      event "Connect Joystick": Value Change {
        n45 = event-data() -> ()  [unwired: 1 in, 6 out]
        n46 = call <vilib>:"Initialize Joystick.vi"("device index"=0) -> ("error out"=w94:errorcluster, "device ID"=w96:refnum<k1>)  [unwired: 9 in]
        n47 = Unbundle By Name(w94) -> ("status"=w93:bool)
        n48 = Not(x=w93) -> (.not. x?=w92:bool)
        n49 = Bundle By Name(cluster=w97, "device ID"=w96, "Joystick Connected"=w92) -> (w95:T27)
      }
      event User Event {
        n50 = event-data() -> ("Msg Type"=w105:T29, "RDS Msg"=w103:refnum<class "RDS Message.lvclass">)  [unwired: 1 in]
        n51 = case shown="\"RDS Message\", Default" w105 {
          tunnel: w111 -> [w119 w266]
          tunnel: w110 -> [_ w267]
          tunnel: [FALSE TRUE] -> w109
          tunnel: [w120 w266] -> w108
          tunnel: [w118 w265] -> w107
          tunnel: w106 -> [w117 w265]
          tunnel: w104 -> [_ w264]
          tunnel: w103 -> [w116 _]
          tunnel: [w113 w263] -> w102
          tunnel: w101 -> [_ w263]
          frame "RDS Message", Default {
            n52 = call "Read Msg Header ID.vi"("RDS Message in"=w116) -> ("Time Stamp"=w112:timestamp, "Msg ID"=w115:T33, "RDS Message out"=w114:refnum<class "RDS Message.lvclass">)  [unwired: 6 in, 2 out]
            n53 = case shown="\"State_Sample\"" w115 {
              tunnel: [w123 w127 w128 w131 w134 w137 w140 w143 w146 w149 w153 w174 w177 w180 w221 w230 w233 w236 w239 w242 w245 w248 w251 w254 w257 w262] -> w120
              tunnel: w119 -> [w123 w127 w128 w131 w134 w137 w140 w143 w146 w149 w154 w174 w177 w180 w221 w230 w233 w236 w239 w242 w245 w248 w251 w254 w257 w262]
              tunnel: [w124 w126 w129 w132 w135 w138 w141 w144 w147 w150 w160 w175 w178 w181 w208 w231 w234 w237 w240 w243 w246 w249 w252 w255 w258 w261] -> w118
              tunnel: w117 -> [w124 w126 w129 w132 w135 w138 w141 w144 w147 w150 w160 w175 w178 w181 _ w231 w234 w237 w240 w243 w246 w249 w252 w255 w258 w261]
              tunnel: w114 -> [_ _ _ _ _ _ _ _ _ _ w156 _ _ _ w216 _ _ _ _ _ _ _ _ _ _ _]
              tunnel: [w122 w125 w130 w133 w136 w139 w142 w145 w148 w151 w152 w176 w179 w182 w222 w232 w235 w238 w241 w244 w247 w250 w253 w256 w259 w260] -> w113
              tunnel: w112 -> [w122 w125 w130 w133 w136 w139 w142 w145 w148 w151 w152 w176 w179 w182 w222 w232 w235 w238 w241 w244 w247 w250 w253 w256 w259 w260]
              frame "RDS Hello World", Default {
              }
              frame "String Message" {
              }
              frame "AIP_Status" {
              }
              frame "AIP_Command" {
              }
              frame "GPS_Data" {
              }
              frame "MCB_Command" {
              }
              frame "MCB_Status" {
              }
              frame "Compass_Data" {
              }
              frame "Depth_Data" {
              }
              frame "Battery_Data" {
              }
              frame "Controller_Message" {
                n54 = To More Specific Class(target class=refnum<class "Controller Message.lvclass"> refnum ("RDS Child Messages.lvlib:Controller Message.lvclass"), reference=w156) -> (specific class reference=w158:refnum<class "Controller Message.lvclass">)  [unwired: 1 in, 1 out]
                n55 = call "Read Controller Address.vi"("Controller Message in"=w158) -> ("Controller"=w155:T2)  [unwired: 8 in, 2 out]
                n56 = call "Read Controller Message Type.vi"("Controller Message in"=w158) -> ("Controller Message Type"=w157:T34)  [unwired: 8 in, 2 out]
                n57 = case shown="\"Shore Remote Control\"" w155 {
                  tunnel: w157 -> [_ w165]
                  tunnel: w154 -> [w161 w164]
                  tunnel: [w161 w163] -> w153
                  tunnel: w152 -> [_ w162]
                  frame "Idle", Default {
                  }
                  frame "Shore Remote Control" {
                    n58 = case shown="\"Control Relinquish Request\", Default" w165 {
                      tunnel: w164 -> [w166 w169 w173]
                      tunnel: [w166 w167 w171] -> w163
                      tunnel: w162 -> [_ _ w170]
                      frame "Control Relinquish Request", Default {
                        # "not for us"
                      }
                      frame "Control Relinquish Command" {
                        n59 = Bundle By Name(cluster=w169, "iHasControl"=FALSE) -> (w167:T27)
                      }
                      frame "Control Granted" {
                        n60 = Bundle By Name(cluster=w173, "iHasControl"=TRUE, "controlTimer"=w170) -> (w171:T27)
                      }
                    }
                  }
                }
              }
              frame "Set_Mag_Dev" {
              }
              frame "BTB_Shutdown" {
              }
              frame "State_Sample_Request" {
              }
              frame "State_Sample" {
                n61 = To More Specific Class(target class=refnum<class "State Sample Message.lvclass"> refnum ("RDS Child Messages.lvlib:State Sample Message.lvclass"), reference=w216) -> (specific class reference=w214:refnum<class "State Sample Message.lvclass">)  [unwired: 1 in, 1 out]
                n62 = call "Read State Sample Message.vi"("State Sample Message in"=w214) -> ("State Sample"=w208:refnum<class "RDS State.lvclass">)  [unwired: 8 in, 2 out]
                n63 = call "SR_Gen_Overview.vi"("State Sample"=w208) -> ("Overview"=→"Overview":T4, "State Sample Out"=w210:refnum<class "RDS State.lvclass">)  [unwired: 9 in]
                n64 = local read "Track"() -> (w189:cluster{"Long":dbl[], "Lat":dbl[]})
                n65 = call "Read Robodolf Controller State.vi"("RDS State in"=w208) -> ("Controller State"=→"RoboDolf State":T2)  [unwired: 8 in, 2 out]
                n66 = call "Read Battery Pack Info.vi"("RDS State in"=w208) -> ("Battery Pack Info"=w197:T22)  [unwired: 8 in, 2 out]
                "Battery Pack Info" <- w197
                n67 = call "Read AIP Status.vi"("RDS State in"=w208) -> ("AIP Status"=w218:T9)  [unwired: 8 in, 2 out]
                "AIP Status" <- w218
                n68 = call "Read Helm Status.vi"("RDS State in"=w208) -> ("Helm Status"=w202:T12)  [unwired: 8 in, 2 out]
                "Helm Status" <- w202
                n69 = call "Read Mission Controller State.vi"("RDS State in"=w208) -> ("Mission Controller State"=→"Mission Controller State":T17)  [unwired: 8 in, 2 out]
                n70 = call "Read Port Motor Status.vi"("RDS State in"=w208) -> ("Port Motor Data"=w207:T24)  [unwired: 8 in, 2 out]
                "Port Motor Data" <- w207
                n71 = call "Read STBD Motor Status.vi"("RDS State in"=w208) -> ("STBD Motor"=w205:T24)  [unwired: 8 in, 2 out]
                "STBD Motor" <- w205
                n72 = call "Read raw Compass Data.vi"("RDS State in"=w208) -> ("Compass Data"=→"Compass Data":T5)  [unwired: 8 in, 2 out]
                n73 = call "Read GPRMC-data.vi"("RDS State in"=w208) -> ("GPRMC-data"=w190:T6)  [unwired: 8 in, 2 out]
                "GPRMC-data" <- w190
                n74 = Unbundle By Name(w190) -> ("GPS Longitude"=w188:dbl, "GPS Latitude"=w187:dbl)
                n75 = Unbundle By Name(w202) -> ("Heading Command Control.Heading"=→"Rudder Chart":sgl, "Heading Command Control.Heading"=w200:sgl, "Current Heading"=w199:dbl)
                n76 = in-place {
                  in-place-border: w188 -> [w228]
                  in-place-border: w187 -> [w225]
                  n77 = in-place-cluster #5(w189) -> ("Long"=w229:dbl[], "Lat"=w226:dbl[])
                  n78 = Build Array (concatenate)(w229, w228) -> (w227:dbl[])
                  n79 = Build Array (concatenate)(w226, w225) -> (w224:dbl[])
                  n80 = in-place-cluster #5("Long"=w227, "Lat"=w224) -> (w185:cluster{"Long":dbl[], "Lat":dbl[]})
                }
                n81 = call "SR_Thermal.vi"("State Sample"=w210) -> ("Thermal"=→"Thermal":T25, "Thermal Points"=→"Thermal WF":sgl[])  [unwired: 8 in, 1 out]
                n82 = Unbundle By Name(w207) -> ("Motor Power"=w206:i16)
                n83 = Unbundle By Name(w205) -> ("Motor Power"=w204:i16)
                n84 = Unbundle By Name(w197) -> ("Pack Current"=w196:sgl, "Pack Capacity"=w195:sgl, "Max Cell Voltage"=w193:sgl, "Min Cell Voltage"=w192:sgl)
                n85 = control-ref of="AIP controls"() -> (w217:refnum<vi>)
                n86 = local read "XY Graph"() -> (w186:cluster{dbl[], dbl[]}[])
                n87 = Bundle("Motor Power"=w206, "Motor Power"=w204) -> (→"Throttles":cluster{"Motor Power":i16, "Motor Power":i16})  [unwired: 1 in]
                n88 = Bundle("Pack Current"=w196, "Pack Capacity"=w195) -> (→"Pow Cap Chart":cluster{"Pack Current":sgl, "Pack Capacity":sgl})  [unwired: 1 in]
                n89 = Bundle("Max Cell Voltage"=w193, "Min Cell Voltage"=w192) -> (→"Voltage Chart":T21)  [unwired: 1 in]
                n90 = call "GUI AIP.vi"("AIP Status"=w218, "Cluster in"=w217) -> ()  [unwired: 10 in]
                n91 = Bundle("Heading"=w200, "Current Heading"=w199) -> (→"Hdng Chart":cluster{"Heading":sgl, "Current Heading":dbl})  [unwired: 1 in]
                n92 = in-place {
                  in-place-border: w185 -> [w223]
                  n93 = in-place-array #6(w186, 0) -> ()  [unwired: 1 out]
                  n94 = in-place-array #6(w223) -> (w183:cluster{dbl[], dbl[]}[])  [unwired: 1 out]
                }
                n95 = local write "Track"(w185) -> ()
                n96 = local write "XY Graph"(w183) -> ()
              }
              frame "PID_Gains_Set" {
              }
              frame "Helm_Limiter_Set" {
              }
              frame "Helm_Heading_Command" {
              }
              frame "Helm_Steering_Command" {
              }
              frame "Helm_Status" {
              }
              frame "AIP_Set_Min_Depth" {
              }
              frame "Mission_Controller_State" {
              }
              frame "Mission_Upload" {
              }
              frame "Mission_Set_Op_and_Run" {
              }
              frame "Mission_Settings_Set" {
              }
              frame "Contoller_State" {
              }
            }
          }
          frame "Shutdown" {
            n97 = Unregister For Events(event registration refnum=w267) -> ()  [unwired: 1 in, 1 out]
            n98 = Destroy User Event(user event=w264) -> ()  [unwired: 1 in, 1 out]
          }
        }
      }
      event "btn_upload_mission": Value Change {
        n99 = event-data() -> ()  [unwired: 1 in, 6 out]
        n100 = Two Button Dialog(message="Are  you sure you want to upload the buffer mission to the RoboDolf?") -> (T button?=w270:bool)  [unwired: 2 in]
        n101 = case shown="True" w270 {
          tunnel: w269 -> [_ w275]
          frame False {
          }
          frame True {
            n102 = local read "Mission Buffer"() -> (w277:T19[])
            n103 = call "Pack Mission Upload Message.vi"("Test Mission"=w277) -> ("Mission Upload Message out"=w276:refnum<class "Mission Upload Message.lvclass">)  [unwired: 10 in]
            n104 = Generate User Event(user event=w275, event data cluster=w276) -> ()  [unwired: 2 in, 2 out]
          }
        }
      }
      event "btn_save_track": Value Change {
        n105 = event-data() -> ()  [unwired: 1 in, 6 out]
        n106 = local read "Track"() -> (w279:cluster{"Long":dbl[], "Lat":dbl[]})
        n107 = Write to Binary File(data=w279) -> (error out=w278:errorcluster)  [unwired: 5 in, 2 out]
        n108 = call <vilib>:"Clear Errors.vi"("error in (no error)"=w278) -> ()  [unwired: 5 in, 2 out]
      }
      event "btn_mission_maker": Value Change {
        n109 = event-data() -> ()  [unwired: 1 in, 6 out]
        n110 = Current VI's Path() -> (path=w284:path)
        n111 = Strip Path(path=w284) -> (stripped path=w283:path)  [unwired: 1 out]
        n112 = Build Path(base path=w283, name or relative path="SR_M-Mission_Util.vi") -> (appended path=w296:path)
        n113 = Open VI Reference(vi path=w296) -> (vi reference=w295:refnum<vi>, error out=w291:errorcluster)  [unwired: 5 in]
        n114 = invoke class="VI" method="FP.Open"(reference=w295, error in=w291, "Activate"=TRUE ("Activate?"), "State"=T32."Standard") -> (reference out=w292:refnum<vi>, error out=w290:errorcluster)  [unwired: 1 in, 3 out]
        n115 = invoke class="VI" method="Run VI"(reference=w292, error in=w290, "Wait until done"=FALSE ("Wait Until Done"), "Auto Dispose Ref"=FALSE ("Auto Dispose Reference")) -> (reference out=w287:refnum<vi>, error out=w286:errorcluster)  [unwired: 1 in, 3 out]
        n116 = Close Reference(reference=w287, error in (no error)=w286) -> (error out=w285:errorcluster)
        n117 = call <vilib>:"Simple Error Handler.vi"("error in (no error)"=w285) -> ()  [unwired: 4 in, 5 out]
      }
      event "Shutdown Safety": Value Change {
        n118 = event-data() -> ("NewVal"=w301:bool)  [unwired: 1 in, 5 out]
        n119 = case shown="False" w301 {
          frame True {
            n120 = property on="btn-emergency-shutdown" class="Bool"("DisabledEnum"=T26."Enabled" ("Disabled")) -> ()  [unwired: 2 in, 2 out]
          }
          frame False {
            n121 = property on="btn-emergency-shutdown" class="Bool"("DisabledEnum"=T26."Disabled and Grayed Out" ("Disabled")) -> ()  [unwired: 2 in, 2 out]
          }
        }
      }
      event "btn-emergency-shutdown": Value Change {
        n122 = event-data() -> ()  [unwired: 1 in, 6 out]
        n123 = Two Button Dialog(message="WARNING!\n\nAre you sure you want to shutdown the battery?\n\nSystem will cut power in 60 seconds if you click yes ") -> (T button?=w309:bool)  [unwired: 2 in]
        n124 = case shown="True" w309 {
          tunnel: w307 -> [_ w313]
          frame False {
          }
          frame True {
            n125 = Get Date/Time In Seconds() -> (seconds since 1Jan1904=w316:timestamp)
            n126 = call "Write Msg Header.vi"("Sender Name"="mr. testy", "Time Stamp"=w316, "Msg ID"=RDS_Message_ID."BTB_Shutdown") -> ("RDS Message out"=w314:refnum<class "RDS Message.lvclass">)  [unwired: 7 in, 1 out]
            n127 = Generate User Event(user event=w313, event data cluster=w314) -> ()  [unwired: 2 in, 2 out]
          }
        }
      }
      event "btn_set_op_run": Value Change {
        n128 = event-data() -> ()  [unwired: 1 in, 6 out]
        n129 = call "Pack SetOp And Run.vi"("MissionOp Index"="MissionOp Index") -> ("Mission Set Op Index and Run Msg out"=w319:refnum<class "Mission Set Op Index and Run Msg.lvclass">)  [unwired: 10 in]
        n130 = Generate User Event(user event=w318, event data cluster=w319) -> ()  [unwired: 2 in, 2 out]
      }
      event "btn_Turneffe": Value Change {
        n131 = event-data() -> ()  [unwired: 1 in, 6 out]
        n132 = property on="XY Graph" class="XYGraph (strict)"("XScale.Maximum"=-87.79375 ("X Scale.Range:Maximum"), "XScale.Minimum"=-87.841656 ("X Scale.Range:Maximum"), "YScale.Maximum"=17.329 ("X Scale.Range:Maximum"), "YScale.Minimum"=17.254657 ("X Scale.Range:Maximum")) -> ()  [unwired: 2 in, 2 out]
      }
      event "btn_beach1": Value Change {
        n133 = event-data() -> ()  [unwired: 1 in, 6 out]
        n134 = property on="XY Graph" class="XYGraph (strict)"("XScale.Maximum"=-87.8089 ("X Scale.Range:Maximum"), "XScale.Minimum"=-87.811885 ("X Scale.Range:Maximum"), "YScale.Maximum"=17.284307 ("X Scale.Range:Maximum"), "YScale.Minimum"=17.27641 ("X Scale.Range:Maximum")) -> ()  [unwired: 2 in, 2 out]
      }
      event "btn_beach 2": Value Change {
        n135 = event-data() -> ()  [unwired: 1 in, 6 out]
        n136 = property on="XY Graph" class="XYGraph (strict)"("XScale.Maximum"=-87.802141 ("X Scale.Range:Maximum"), "XScale.Minimum"=-87.80894 ("X Scale.Range:Maximum"), "YScale.Maximum"=17.30965 ("X Scale.Range:Maximum"), "YScale.Minimum"=17.297963 ("X Scale.Range:Maximum")) -> ()  [unwired: 2 in, 2 out]
      }
      event "btn_gains set": Value Change {
        n137 = event-data() -> ()  [unwired: 1 in, 6 out]
        n138 = Get Date/Time In Seconds() -> (seconds since 1Jan1904=w348:timestamp)
        n139 = call "Write Msg Header.vi"("Sender Name"="mr. testy", "Time Stamp"=w348, "Msg ID"=RDS_Message_ID."PID_Gains_Set", "RDS Message in"=refnum<class "PID Gains Set Message.lvclass"> refnum ("RDS Child Messages.lvlib:PID Gains Set Message.lvclass")) -> ("RDS Message out"=w351:refnum<class "PID Gains Set Message.lvclass">)  [unwired: 6 in, 1 out]
        n140 = call "Write Gains Message.vi"("Gains"="Gains", "PID Gains Set Message in"=w351) -> ("PID Gains Set Message out"=w345:refnum<class "PID Gains Set Message.lvclass">)  [unwired: 8 in, 1 out]
        n141 = Generate User Event(user event=w346, event data cluster=w345) -> ()  [unwired: 2 in, 2 out]
      }
      event "btn_set_mag_dev": Value Change {
        n142 = event-data() -> ()  [unwired: 1 in, 6 out]
        n143 = call "Pack Mag Dev Msg.vi"("Compass Mag Dev"="Compass Mag Dev") -> ("Set Mag Dev Message out"=w356:refnum<class "Set Mag Dev Message.lvclass">)  [unwired: 10 in]
        n144 = Generate User Event(user event=w357, event data cluster=w356) -> ()  [unwired: 2 in, 2 out]
      }
      event "btn_Send-Steer": Value Change {
        n145 = event-data() -> ()  [unwired: 1 in, 6 out]
        n146 = Get Date/Time In Seconds() -> (seconds since 1Jan1904=w364:timestamp)
        n147 = call "Write Msg Header.vi"("Sender Name"="mr. testy", "Time Stamp"=w364, "Msg ID"=RDS_Message_ID."Helm_Steering_Command", "RDS Message in"=refnum<class "Steering Command.lvclass"> refnum ("RDS Child Messages.lvlib:Steering Command.lvclass")) -> ("RDS Message out"=w366:refnum<class "Steering Command.lvclass">)  [unwired: 6 in, 1 out]
        n148 = call "Write Steering Command Message.vi"("Steering Command Control"="Steering Command", "Steering Command in"=w366) -> ("Steering Command out"=w362:refnum<class "Steering Command.lvclass">)  [unwired: 8 in, 1 out]
        n149 = Generate User Event(user event=w369, event data cluster=w362) -> ()  [unwired: 2 in, 2 out]
      }
      event "btn_mission_ReqControl": Value Change {
        n150 = event-data() -> ()  [unwired: 1 in, 6 out]
        n151 = Get Date/Time In Seconds() -> (seconds since 1Jan1904=w376:timestamp)
        n152 = call "Write Msg Header.vi"("Sender Name"="mr. testy", "Time Stamp"=w376, "Msg ID"=RDS_Message_ID."Controller_Message", "RDS Message in"=refnum<class "Controller Message.lvclass"> refnum ("RDS Child Messages.lvlib:Controller Message.lvclass")) -> ("error out"=w379:errorcluster, "RDS Message out"=w380:refnum<class "Controller Message.lvclass">)  [unwired: 6 in]
        n153 = call "Write Controller Message Type.vi"("error in (no error)"=w379, "Controller Message Type"=Controller_Message_Type."Control Request", "Controller Message in"=w380) -> ("error out"=w383:errorcluster, "Controller Message out"=w382:refnum<class "Controller Message.lvclass">)  [unwired: 7 in]
        n154 = call "Write Controller Address.vi"("error in (no error)"=w383, "Controller"=Controller."Mission Control", "Controller Message in"=w382) -> ("Controller Message out"=w373:refnum<class "Controller Message.lvclass">)  [unwired: 7 in, 1 out]
        n155 = Generate User Event(user event=w374, event data cluster=w373) -> ()  [unwired: 2 in, 2 out]
      }
      event "btn_mission_Relinquish": Value Change {
        n156 = event-data() -> ()  [unwired: 1 in, 6 out]
        n157 = Get Date/Time In Seconds() -> (seconds since 1Jan1904=w391:timestamp)
        n158 = call "Write Msg Header.vi"("Sender Name"="mr. testy", "Time Stamp"=w391, "Msg ID"=RDS_Message_ID."Controller_Message", "RDS Message in"=refnum<class "Controller Message.lvclass"> refnum ("RDS Child Messages.lvlib:Controller Message.lvclass")) -> ("error out"=w394:errorcluster, "RDS Message out"=w395:refnum<class "Controller Message.lvclass">)  [unwired: 6 in]
        n159 = call "Write Controller Message Type.vi"("error in (no error)"=w394, "Controller Message Type"=Controller_Message_Type."Control Relinquish Request", "Controller Message in"=w395) -> ("error out"=w398:errorcluster, "Controller Message out"=w397:refnum<class "Controller Message.lvclass">)  [unwired: 7 in]
        n160 = call "Write Controller Address.vi"("error in (no error)"=w398, "Controller"=Controller."Mission Control", "Controller Message in"=w397) -> ("Controller Message out"=w389:refnum<class "Controller Message.lvclass">)  [unwired: 7 in, 1 out]
        n161 = Generate User Event(user event=w388, event data cluster=w389) -> ()  [unwired: 2 in, 2 out]
      }
      event "btn_send settings": Value Change {
        n162 = event-data() -> ()  [unwired: 1 in, 6 out]
        n163 = call "Pack Mission Mission Settings Message.vi"("Mission Controller Settings"="Mission Controller Settings") -> ("Set Mission Controller Settings Message out"=w403:refnum<class "Set Mission Controller Settings Message.lvclass">)  [unwired: 10 in]
        n164 = Generate User Event(user event=w404, event data cluster=w403) -> ()  [unwired: 2 in, 2 out]
      }
      event "btn_set_aip_min_depth": Value Change {
        n165 = event-data() -> ()  [unwired: 1 in, 6 out]
        n166 = Get Date/Time In Seconds() -> (seconds since 1Jan1904=w412:timestamp)
        n167 = call "Write Msg Header.vi"("Sender Name"="mr. testy", "Time Stamp"=w412, "Msg ID"=RDS_Message_ID."AIP_Set_Min_Depth", "RDS Message in"=refnum<class "AIP Set Min Depth Message.lvclass"> refnum ("RDS Child Messages.lvlib:AIP Set Min Depth Message.lvclass")) -> ("RDS Message out"=w415:refnum<class "AIP Set Min Depth Message.lvclass">)  [unwired: 6 in, 1 out]
        n168 = call "Write Min Depth Message.vi"("Min Depth"="AIP Min Depth", "AIP Set Min Depth Message in"=w415) -> ("AIP Set Min Depth Message out"=w410:refnum<class "AIP Set Min Depth Message.lvclass">)  [unwired: 8 in, 1 out]
        n169 = Generate User Event(user event=w409, event data cluster=w410) -> ()  [unwired: 2 in, 2 out]
      }
      event "btn_limiter_set": Value Change {
        n170 = event-data() -> ()  [unwired: 1 in, 6 out]
        n171 = Get Date/Time In Seconds() -> (seconds since 1Jan1904=w423:timestamp)
        n172 = call "Write Msg Header.vi"("Sender Name"="mr. testy", "Time Stamp"=w423, "Msg ID"=RDS_Message_ID."Helm_Limiter_Set", "RDS Message in"=refnum<class "Helm Limiter Msg.lvclass"> refnum ("RDS Child Messages.lvlib:Helm Limiter Msg.lvclass")) -> ("RDS Message out"=w426:refnum<class "Helm Limiter Msg.lvclass">)  [unwired: 6 in, 1 out]
        n173 = call "Write Limiter Msg.vi"("Limiter"="Limter", "Helm Limiter Msg in"=w426) -> ("Helm Limiter Msg out"=w420:refnum<class "Helm Limiter Msg.lvclass">)  [unwired: 8 in, 1 out]
        n174 = Generate User Event(user event=w421, event data cluster=w420) -> ()  [unwired: 2 in, 2 out]
      }
      event "AIP Stow": Value Change {
        n175 = event-data() -> ()  [unwired: 1 in, 6 out]
        n176 = Get Date/Time In Seconds() -> (seconds since 1Jan1904=w436:timestamp)
        n177 = call "Write Msg Header.vi"("Sender Name"="mr. testy", "Time Stamp"=w436, "Msg ID"=RDS_Message_ID."AIP_Command", "RDS Message in"=refnum<class "AIP Command.lvclass"> refnum ("RDS Child Messages.lvlib:AIP Command.lvclass")) -> ("RDS Message out"=w437:refnum<class "AIP Command.lvclass">)  [unwired: 6 in, 1 out]
        n178 = call "Write AIP.vi"("AIP Command"=AIP_Command_Control."Stow", "AIP Deploy Command in"=w437) -> ("AIP Deploy Command out"=w432:refnum<class "AIP Command.lvclass">)  [unwired: 8 in, 1 out]
        n179 = Generate User Event(user event=w433, event data cluster=w432) -> ()  [unwired: 2 in, 2 out]
      }
      event "AIP Deploy": Value Change {
        n180 = event-data() -> ()  [unwired: 1 in, 6 out]
        n181 = Get Date/Time In Seconds() -> (seconds since 1Jan1904=w447:timestamp)
        n182 = call "Write Msg Header.vi"("Sender Name"="mr. testy", "Time Stamp"=w447, "Msg ID"=RDS_Message_ID."AIP_Command", "RDS Message in"=refnum<class "AIP Command.lvclass"> refnum ("RDS Child Messages.lvlib:AIP Command.lvclass")) -> ("RDS Message out"=w448:refnum<class "AIP Command.lvclass">)  [unwired: 6 in, 1 out]
        n183 = call "Write AIP.vi"("AIP Command"=AIP_Command_Control."Deploy", "AIP Deploy Command in"=w448) -> ("AIP Deploy Command out"=w443:refnum<class "AIP Command.lvclass">)  [unwired: 8 in, 1 out]
        n184 = Generate User Event(user event=w444, event data cluster=w443) -> ()  [unwired: 2 in, 2 out]
      }
      event "AIP Stop": Value Change {
        n185 = event-data() -> ()  [unwired: 1 in, 6 out]
        n186 = Get Date/Time In Seconds() -> (seconds since 1Jan1904=w458:timestamp)
        n187 = call "Write Msg Header.vi"("Sender Name"="mr. testy", "Time Stamp"=w458, "Msg ID"=RDS_Message_ID."AIP_Command", "RDS Message in"=refnum<class "AIP Command.lvclass"> refnum ("RDS Child Messages.lvlib:AIP Command.lvclass")) -> ("RDS Message out"=w459:refnum<class "AIP Command.lvclass">)  [unwired: 6 in, 1 out]
        n188 = call "Write AIP.vi"("AIP Command"=AIP_Command_Control."Stop", "AIP Deploy Command in"=w459) -> ("AIP Deploy Command out"=w454:refnum<class "AIP Command.lvclass">)  [unwired: 8 in, 1 out]
        n189 = Generate User Event(user event=w455, event data cluster=w454) -> ()  [unwired: 2 in, 2 out]
      }
      event "AIP JD FP": Value Change {
        n190 = event-data() -> ()  [unwired: 1 in, 6 out]
        n191 = Get Date/Time In Seconds() -> (seconds since 1Jan1904=w469:timestamp)
        n192 = call "Write Msg Header.vi"("Sender Name"="mr. testy", "Time Stamp"=w469, "Msg ID"=RDS_Message_ID."AIP_Command", "RDS Message in"=refnum<class "AIP Command.lvclass"> refnum ("RDS Child Messages.lvlib:AIP Command.lvclass")) -> ("RDS Message out"=w470:refnum<class "AIP Command.lvclass">)  [unwired: 6 in, 1 out]
        n193 = call "Write AIP.vi"("AIP Command"=AIP_Command_Control."Jog Deploy FP", "AIP Deploy Command in"=w470) -> ("AIP Deploy Command out"=w465:refnum<class "AIP Command.lvclass">)  [unwired: 8 in, 1 out]
        n194 = Generate User Event(user event=w466, event data cluster=w465) -> ()  [unwired: 2 in, 2 out]
      }
      event "AIP D FP": Value Change {
        n195 = event-data() -> ()  [unwired: 1 in, 6 out]
        n196 = Get Date/Time In Seconds() -> (seconds since 1Jan1904=w480:timestamp)
        n197 = call "Write Msg Header.vi"("Sender Name"="mr. testy", "Time Stamp"=w480, "Msg ID"=RDS_Message_ID."AIP_Command", "RDS Message in"=refnum<class "AIP Command.lvclass"> refnum ("RDS Child Messages.lvlib:AIP Command.lvclass")) -> ("RDS Message out"=w481:refnum<class "AIP Command.lvclass">)  [unwired: 6 in, 1 out]
        n198 = call "Write AIP.vi"("AIP Command"=AIP_Command_Control."Deploy FP", "AIP Deploy Command in"=w481) -> ("AIP Deploy Command out"=w476:refnum<class "AIP Command.lvclass">)  [unwired: 8 in, 1 out]
        n199 = Generate User Event(user event=w477, event data cluster=w476) -> ()  [unwired: 2 in, 2 out]
      }
      event "AIP D FS": Value Change {
        n200 = event-data() -> ()  [unwired: 1 in, 6 out]
        n201 = Get Date/Time In Seconds() -> (seconds since 1Jan1904=w491:timestamp)
        n202 = call "Write Msg Header.vi"("Sender Name"="mr. testy", "Time Stamp"=w491, "Msg ID"=RDS_Message_ID."AIP_Command", "RDS Message in"=refnum<class "AIP Command.lvclass"> refnum ("RDS Child Messages.lvlib:AIP Command.lvclass")) -> ("RDS Message out"=w492:refnum<class "AIP Command.lvclass">)  [unwired: 6 in, 1 out]
        n203 = call "Write AIP.vi"("AIP Command"=AIP_Command_Control."Deploy FS", "AIP Deploy Command in"=w492) -> ("AIP Deploy Command out"=w487:refnum<class "AIP Command.lvclass">)  [unwired: 8 in, 1 out]
        n204 = Generate User Event(user event=w488, event data cluster=w487) -> ()  [unwired: 2 in, 2 out]
      }
      event "AIP S FS": Value Change {
        n205 = event-data() -> ()  [unwired: 1 in, 6 out]
        n206 = Get Date/Time In Seconds() -> (seconds since 1Jan1904=w502:timestamp)
        n207 = call "Write Msg Header.vi"("Sender Name"="mr. testy", "Time Stamp"=w502, "Msg ID"=RDS_Message_ID."AIP_Command", "RDS Message in"=refnum<class "AIP Command.lvclass"> refnum ("RDS Child Messages.lvlib:AIP Command.lvclass")) -> ("RDS Message out"=w503:refnum<class "AIP Command.lvclass">)  [unwired: 6 in, 1 out]
        n208 = call "Write AIP.vi"("AIP Command"=AIP_Command_Control."Stow FS", "AIP Deploy Command in"=w503) -> ("AIP Deploy Command out"=w498:refnum<class "AIP Command.lvclass">)  [unwired: 8 in, 1 out]
        n209 = Generate User Event(user event=w499, event data cluster=w498) -> ()  [unwired: 2 in, 2 out]
      }
      event "AIP S FP": Value Change {
        n210 = event-data() -> ()  [unwired: 1 in, 6 out]
        n211 = Get Date/Time In Seconds() -> (seconds since 1Jan1904=w513:timestamp)
        n212 = call "Write Msg Header.vi"("Sender Name"="mr. testy", "Time Stamp"=w513, "Msg ID"=RDS_Message_ID."AIP_Command", "RDS Message in"=refnum<class "AIP Command.lvclass"> refnum ("RDS Child Messages.lvlib:AIP Command.lvclass")) -> ("RDS Message out"=w514:refnum<class "AIP Command.lvclass">)  [unwired: 6 in, 1 out]
        n213 = call "Write AIP.vi"("AIP Command"=AIP_Command_Control."Stow FP", "AIP Deploy Command in"=w514) -> ("AIP Deploy Command out"=w509:refnum<class "AIP Command.lvclass">)  [unwired: 8 in, 1 out]
        n214 = Generate User Event(user event=w510, event data cluster=w509) -> ()  [unwired: 2 in, 2 out]
      }
      event "AIP S AP": Value Change {
        n215 = event-data() -> ()  [unwired: 1 in, 6 out]
        n216 = Get Date/Time In Seconds() -> (seconds since 1Jan1904=w524:timestamp)
        n217 = call "Write Msg Header.vi"("Sender Name"="mr. testy", "Time Stamp"=w524, "Msg ID"=RDS_Message_ID."AIP_Command", "RDS Message in"=refnum<class "AIP Command.lvclass"> refnum ("RDS Child Messages.lvlib:AIP Command.lvclass")) -> ("RDS Message out"=w525:refnum<class "AIP Command.lvclass">)  [unwired: 6 in, 1 out]
        n218 = call "Write AIP.vi"("AIP Command"=AIP_Command_Control."Stow AP", "AIP Deploy Command in"=w525) -> ("AIP Deploy Command out"=w520:refnum<class "AIP Command.lvclass">)  [unwired: 8 in, 1 out]
        n219 = Generate User Event(user event=w521, event data cluster=w520) -> ()  [unwired: 2 in, 2 out]
      }
      event "AIP S AS": Value Change {
        n220 = event-data() -> ()  [unwired: 1 in, 6 out]
        n221 = Get Date/Time In Seconds() -> (seconds since 1Jan1904=w535:timestamp)
        n222 = call "Write Msg Header.vi"("Sender Name"="mr. testy", "Time Stamp"=w535, "Msg ID"=RDS_Message_ID."AIP_Command", "RDS Message in"=refnum<class "AIP Command.lvclass"> refnum ("RDS Child Messages.lvlib:AIP Command.lvclass")) -> ("RDS Message out"=w536:refnum<class "AIP Command.lvclass">)  [unwired: 6 in, 1 out]
        n223 = call "Write AIP.vi"("AIP Command"=AIP_Command_Control."Stow AS", "AIP Deploy Command in"=w536) -> ("AIP Deploy Command out"=w531:refnum<class "AIP Command.lvclass">)  [unwired: 8 in, 1 out]
        n224 = Generate User Event(user event=w532, event data cluster=w531) -> ()  [unwired: 2 in, 2 out]
      }
      event "AIP D AP": Value Change {
        n225 = event-data() -> ()  [unwired: 1 in, 6 out]
        n226 = Get Date/Time In Seconds() -> (seconds since 1Jan1904=w546:timestamp)
        n227 = call "Write Msg Header.vi"("Sender Name"="mr. testy", "Time Stamp"=w546, "Msg ID"=RDS_Message_ID."AIP_Command", "RDS Message in"=refnum<class "AIP Command.lvclass"> refnum ("RDS Child Messages.lvlib:AIP Command.lvclass")) -> ("RDS Message out"=w547:refnum<class "AIP Command.lvclass">)  [unwired: 6 in, 1 out]
        n228 = call "Write AIP.vi"("AIP Command"=AIP_Command_Control."Deploy AP", "AIP Deploy Command in"=w547) -> ("AIP Deploy Command out"=w542:refnum<class "AIP Command.lvclass">)  [unwired: 8 in, 1 out]
        n229 = Generate User Event(user event=w543, event data cluster=w542) -> ()  [unwired: 2 in, 2 out]
      }
      event "AIP D FP 4": Value Change {
        n230 = event-data() -> ()  [unwired: 1 in, 6 out]
        n231 = Get Date/Time In Seconds() -> (seconds since 1Jan1904=w557:timestamp)
        n232 = call "Write Msg Header.vi"("Sender Name"="mr. testy", "Time Stamp"=w557, "Msg ID"=RDS_Message_ID."AIP_Command", "RDS Message in"=refnum<class "AIP Command.lvclass"> refnum ("RDS Child Messages.lvlib:AIP Command.lvclass")) -> ("RDS Message out"=w558:refnum<class "AIP Command.lvclass">)  [unwired: 6 in, 1 out]
        n233 = call "Write AIP.vi"("AIP Command"=AIP_Command_Control."Deploy AS", "AIP Deploy Command in"=w558) -> ("AIP Deploy Command out"=w553:refnum<class "AIP Command.lvclass">)  [unwired: 8 in, 1 out]
        n234 = Generate User Event(user event=w554, event data cluster=w553) -> ()  [unwired: 2 in, 2 out]
      }
      event "AIP JD FS": Value Change {
        n235 = event-data() -> ()  [unwired: 1 in, 6 out]
        n236 = Get Date/Time In Seconds() -> (seconds since 1Jan1904=w568:timestamp)
        n237 = call "Write Msg Header.vi"("Sender Name"="mr. testy", "Time Stamp"=w568, "Msg ID"=RDS_Message_ID."AIP_Command", "RDS Message in"=refnum<class "AIP Command.lvclass"> refnum ("RDS Child Messages.lvlib:AIP Command.lvclass")) -> ("RDS Message out"=w569:refnum<class "AIP Command.lvclass">)  [unwired: 6 in, 1 out]
        n238 = call "Write AIP.vi"("AIP Command"=AIP_Command_Control."Jog Deploy FS", "AIP Deploy Command in"=w569) -> ("AIP Deploy Command out"=w564:refnum<class "AIP Command.lvclass">)  [unwired: 8 in, 1 out]
        n239 = Generate User Event(user event=w565, event data cluster=w564) -> ()  [unwired: 2 in, 2 out]
      }
      event "AIP JD AS": Value Change {
        n240 = event-data() -> ()  [unwired: 1 in, 6 out]
        n241 = Get Date/Time In Seconds() -> (seconds since 1Jan1904=w579:timestamp)
        n242 = call "Write Msg Header.vi"("Sender Name"="mr. testy", "Time Stamp"=w579, "Msg ID"=RDS_Message_ID."AIP_Command", "RDS Message in"=refnum<class "AIP Command.lvclass"> refnum ("RDS Child Messages.lvlib:AIP Command.lvclass")) -> ("RDS Message out"=w580:refnum<class "AIP Command.lvclass">)  [unwired: 6 in, 1 out]
        n243 = call "Write AIP.vi"("AIP Command"=AIP_Command_Control."Jog Deploy AS", "AIP Deploy Command in"=w580) -> ("AIP Deploy Command out"=w575:refnum<class "AIP Command.lvclass">)  [unwired: 8 in, 1 out]
        n244 = Generate User Event(user event=w576, event data cluster=w575) -> ()  [unwired: 2 in, 2 out]
      }
      event "AIP JD AP": Value Change {
        n245 = event-data() -> ()  [unwired: 1 in, 6 out]
        n246 = Get Date/Time In Seconds() -> (seconds since 1Jan1904=w590:timestamp)
        n247 = call "Write Msg Header.vi"("Sender Name"="mr. testy", "Time Stamp"=w590, "Msg ID"=RDS_Message_ID."AIP_Command", "RDS Message in"=refnum<class "AIP Command.lvclass"> refnum ("RDS Child Messages.lvlib:AIP Command.lvclass")) -> ("RDS Message out"=w591:refnum<class "AIP Command.lvclass">)  [unwired: 6 in, 1 out]
        n248 = call "Write AIP.vi"("AIP Command"=AIP_Command_Control."Jog Deploy AP", "AIP Deploy Command in"=w591) -> ("AIP Deploy Command out"=w586:refnum<class "AIP Command.lvclass">)  [unwired: 8 in, 1 out]
        n249 = Generate User Event(user event=w587, event data cluster=w586) -> ()  [unwired: 2 in, 2 out]
      }
      event "AIP JS FP": Value Change {
        n250 = event-data() -> ()  [unwired: 1 in, 6 out]
        n251 = Get Date/Time In Seconds() -> (seconds since 1Jan1904=w601:timestamp)
        n252 = call "Write Msg Header.vi"("Sender Name"="mr. testy", "Time Stamp"=w601, "Msg ID"=RDS_Message_ID."AIP_Command", "RDS Message in"=refnum<class "AIP Command.lvclass"> refnum ("RDS Child Messages.lvlib:AIP Command.lvclass")) -> ("RDS Message out"=w602:refnum<class "AIP Command.lvclass">)  [unwired: 6 in, 1 out]
        n253 = call "Write AIP.vi"("AIP Command"=AIP_Command_Control."Jog Stow FP", "AIP Deploy Command in"=w602) -> ("AIP Deploy Command out"=w597:refnum<class "AIP Command.lvclass">)  [unwired: 8 in, 1 out]
        n254 = Generate User Event(user event=w598, event data cluster=w597) -> ()  [unwired: 2 in, 2 out]
      }
      event "AIP JS AP": Value Change {
        n255 = event-data() -> ()  [unwired: 1 in, 6 out]
        n256 = Get Date/Time In Seconds() -> (seconds since 1Jan1904=w612:timestamp)
        n257 = call "Write Msg Header.vi"("Sender Name"="mr. testy", "Time Stamp"=w612, "Msg ID"=RDS_Message_ID."AIP_Command", "RDS Message in"=refnum<class "AIP Command.lvclass"> refnum ("RDS Child Messages.lvlib:AIP Command.lvclass")) -> ("RDS Message out"=w613:refnum<class "AIP Command.lvclass">)  [unwired: 6 in, 1 out]
        n258 = call "Write AIP.vi"("AIP Command"=AIP_Command_Control."Jog Stow AP", "AIP Deploy Command in"=w613) -> ("AIP Deploy Command out"=w608:refnum<class "AIP Command.lvclass">)  [unwired: 8 in, 1 out]
        n259 = Generate User Event(user event=w609, event data cluster=w608) -> ()  [unwired: 2 in, 2 out]
      }
      event "AIP JS AS": Value Change {
        n260 = event-data() -> ()  [unwired: 1 in, 6 out]
        n261 = Get Date/Time In Seconds() -> (seconds since 1Jan1904=w623:timestamp)
        n262 = call "Write Msg Header.vi"("Sender Name"="mr. testy", "Time Stamp"=w623, "Msg ID"=RDS_Message_ID."AIP_Command", "RDS Message in"=refnum<class "AIP Command.lvclass"> refnum ("RDS Child Messages.lvlib:AIP Command.lvclass")) -> ("RDS Message out"=w624:refnum<class "AIP Command.lvclass">)  [unwired: 6 in, 1 out]
        n263 = call "Write AIP.vi"("AIP Command"=AIP_Command_Control."Jog Stow AS", "AIP Deploy Command in"=w624) -> ("AIP Deploy Command out"=w619:refnum<class "AIP Command.lvclass">)  [unwired: 8 in, 1 out]
        n264 = Generate User Event(user event=w620, event data cluster=w619) -> ()  [unwired: 2 in, 2 out]
      }
      event "AIP JS FS": Value Change {
        n265 = event-data() -> ()  [unwired: 1 in, 6 out]
        n266 = Get Date/Time In Seconds() -> (seconds since 1Jan1904=w634:timestamp)
        n267 = call "Write Msg Header.vi"("Sender Name"="mr. testy", "Time Stamp"=w634, "Msg ID"=RDS_Message_ID."AIP_Command", "RDS Message in"=refnum<class "AIP Command.lvclass"> refnum ("RDS Child Messages.lvlib:AIP Command.lvclass")) -> ("RDS Message out"=w635:refnum<class "AIP Command.lvclass">)  [unwired: 6 in, 1 out]
        n268 = call "Write AIP.vi"("AIP Command"=AIP_Command_Control."Jog Stow FS", "AIP Deploy Command in"=w635) -> ("AIP Deploy Command out"=w630:refnum<class "AIP Command.lvclass">)  [unwired: 8 in, 1 out]
        n269 = Generate User Event(user event=w631, event data cluster=w630) -> ()  [unwired: 2 in, 2 out]
      }
    }
    "Last Status Message" <- w34
    n270 = Unbundle By Name(w31) -> ("iHasControl"=→"iHasControl":bool, "Joystick Connected"=→"Joystick Connected":bool)
    n271 = Get Date/Time In Seconds() -> (seconds since 1Jan1904=w33:timestamp)
    n272 = Subtract(x=w33, y=w34) -> (x-y=→"Seconds Ago":dbl)
  }
  n273 = while {
    tunnel: w15 -> [w651]
    shift-right: [w648] -> _
    shift-left: refnum<class "RDS Serial Instrument.lvclass"> refnum ("RDS Serial Handler.lvlib:RDS Serial Instrument.lvclass") -> [w650]
    shift-right: [w647] -> _
    shift-left: errorcluster {"status"=FALSE, "code"=0, "source"=""} ("error out") -> [w644]
    tunnel: w10 -> [w643]
    tunnel: w9 -> [w641]
    stop <- w640 stop-if-true
    # "Serial Event Loop. This loop handles three things. The opening and closing of the serial port, the send of serial data, and the receiving of serial data. It forwards received and decoded RDS messages to the Main Event Loop."
    n274 = event shown="[1] <RDS Message>: User Event" {
      selector: w651 -> [_ _ _ w730]
      dyn-events: _ -> [_ _ _ _]
      timeout: 0 -> [_ _ _ _]
      tunnel: [w656 w694 w713 w728] -> w649
      tunnel: w650 -> [w659 w695 w711 w729]
      tunnel: [w652 w690 w712 w722] -> w646
      tunnel: w644 -> [w657 w691 _ w725]
      tunnel: w643 -> [w655 _ _ w721]
      tunnel: w641 -> [_ _ _ w726]
      tunnel: [_ _ _ TRUE] -> w640
      event Timeout {
        # "Do a serial real. Out serial read handler needs to be polled. It has its own timing delays, which is what throttles the serial read"
        n275 = event-data() -> ()  [unwired: 1 in, 1 out]
        n276 = call "RDS Serial Handler Read.vi"("error in (no error)"=w657, "RDS Serial Instrument in"=w659) -> ("error out"=w653:errorcluster, "Data Valid?"=w654:bool, "RDS Serial Frame out"=w658:refnum<class "RDS Serial Frame.lvclass">, "RDS Serial Instrument out"=w656:refnum<class "RDS Serial Instrument.lvclass">)  [unwired: 6 in]
        n277 = case shown="True" w654 {
          tunnel: w658 -> [_ w666]
          tunnel: w655 -> [_ w665]
          tunnel: w653 -> [w660 w663]
          tunnel: [w660 w662] -> w652
          frame False {
            # "Non valid ( i guess i coulda just said invalid) serial packet, so don't do anything"
          }
          frame True {
            # "Valid serial packet"
            n278 = call "RDS Serial Frame Read.vi"("error in (no error)"=w663, "RDS Serial Frame in"=w666) -> ("error out"=w664:errorcluster, "Serial String"=w661:string)  [unwired: 6 in, 2 out]
            n279 = call "Add zero.vi"("error in (no error)"=w664, "String in"=w661) -> ("error out"=w671:errorcluster, "String out"=w670:string)  [unwired: 8 in]
            n280 = call "Handle Transmission.vi"("error in (no error)"=w671, "Stuffed Data"=w670) -> ("error out"=w668:errorcluster, "Transmission valid?"=w669:bool, "Transmission"=w667:string)  [unwired: 7 in]
            n281 = case shown="True" w669 {
              tunnel: w667 -> [_ w681]
              tunnel: w668 -> [w672 w680]
              tunnel: [w672 w674] -> w662
              tunnel: w665 -> [_ w673]
              frame False {
                # "This isn't the end of the transmission, so just run till we get one"
              }
              frame True {
                # "Valid transmission!"
                n282 = call "GZip Decompress.vi"("error in (no error)"=w680, "GZip compressed string"=w681) -> ("error out"=w675:errorcluster, "Decompressed string"=w678:string)  [unwired: 8 in]
                n283 = Unflatten From String(type=refnum<class "RDS Message.lvclass"> refnum ("RDS Child Messages.lvlib:RDS Message.lvclass"), binary string=w678, error in (no error)=w675) -> (value=w677:refnum<class "RDS Message.lvclass">, error out=w676:errorcluster)  [unwired: 2 in, 1 out]
                n284 = case shown="No Error" w676 {
                  selector: w676 -> [w683 _]
                  tunnel: w677 -> [w684 _]
                  tunnel: w673 -> [w687 _]
                  tunnel: [w682 errorcluster {"status"=FALSE, "code"=0, "source"=""} ("error out")] -> w674
                  frame No Error {
                    n285 = Bundle("RDS Shore Remote Msg"=RDS_Q_Message."RDS Message", "RDS Child Messages.lvlib:RDS Message.lvclass"=w684) -> (w686:T36)  [unwired: 1 in]
                    n286 = Generate User Event(user event=w687, event data cluster=w686, error in=w683) -> (error out=w682:errorcluster)  [unwired: 1 in, 1 out]
                  }
                  frame Error {
                  }
                }
              }
            }
          }
        }
      }
      event User Event {
        # "Here we take an RDS Message that has been queued up and blast it over the air!"
        # "Blast an RDS message over the air!"
        n287 = event-data() -> ("RDS Message"=w689:refnum<class "RDS Message.lvclass">)  [unwired: 1 in]
        n288 = Flatten To String(anything=w689, error in (no error)=w691) -> (data string=w693:string, error out=w692:errorcluster)  [unwired: 2 in, 1 out]
        n289 = call "GZip Compress.vi"("error in (no error)"=w692, "Uncompressed string"=w693) -> ("error out"=w698:errorcluster, "GZip compressed string"=w700:string)  [unwired: 7 in, 1 out]
        n290 = String Length(string=w700) -> (length=→"Tx packet  length":i32)
        n291 = call "LSR Make Transmission.vi"("error in (no error)"=w698, "Data String"=w700) -> ("error out"=w697:errorcluster, "Transmission"=w699:string[])  [unwired: 8 in]
        n292 = for {
          tunnel: w699 -> [w710] mode=indexing
          shift-right: [w701] -> w690
          shift-left: w697 -> [w709]
          shift-right: [w704] -> w694
          shift-left: w695 -> [w705]
          n293 = call "Delete Zero.vi"("error in (no error)"=w709, "COBS String in"=w710) -> ("error out"=w706:errorcluster, "String out"=w707:string)  [unwired: 8 in]
          n294 = Get Date/Time In Seconds() -> (seconds since 1Jan1904=w708:timestamp)
          n295 = call "RDS Serial Frame Write.vi"("error in (no error)"=w706, "Time Stamp"=w708, "Serial String"=w707) -> ("error out"=w702:errorcluster, "RDS Serial Frame out"=w703:refnum<class "RDS Serial Frame.lvclass">)  [unwired: 7 in]
          n296 = call "RDS Serial Handler Send Frame.vi"("error in (no error)"=w702, "Serial Frame"=w703, "RDS Serial Instrument in"=w705) -> ("error out"=w701:errorcluster, "RDS Serial Instrument out"=w704:refnum<class "RDS Serial Instrument.lvclass">)  [unwired: 7 in]
        }
      }
      event "Digi Connect": Value Change {
        # "Connect up the serial port"
        n297 = event-data() -> ()  [unwired: 1 in, 1 out]
        n298 = call "LSR Terminal String.vi"() -> ("LSR Term"=w714:string)  [unwired: 11 in]
        n299 = call "RDS Serial Handler Initialize.vi"("Termination Char(s)"=w714, "baud rate (9600)"=u32 115200, "VISA resource name"="Digi Serial Port", "RDS Serial Instrument in"=w711) -> ("error out"=w712:errorcluster, "RDS Serial Instrument out"=w713:refnum<class "RDS Serial Instrument.lvclass">)  [unwired: 6 in]
      }
      event "stop": Value Change {
        # "Send a shut down signal to the main loop"
        n300 = event-data() -> ()  [unwired: 1 in, 1 out]
        n301 = Bundle("RDS Shore Remote Msg"=RDS_Q_Message."Shutdown", "RDS Child Messages.lvlib:RDS Message.lvclass"=refnum<class "RDS Message.lvclass"> refnum) -> (w718:T36)  [unwired: 1 in]
        n302 = Generate User Event(user event=w721, event data cluster=w718) -> ()  [unwired: 2 in, 2 out]
        n303 = Unregister For Events(event registration refnum=w730, error in=w725) -> (error out=w724:errorcluster)
        n304 = flat-sequence {
          tunnel: w726 -> [w732]
          tunnel: w724 -> [_]
          tunnel: [w731] -> w723
          frame #0 {
            # "We want this to run even if there is an error upstream, but we want it to run after the unregister and not before so we chain it still"
            n305 = Destroy User Event(user event=w732) -> (error out=w731:errorcluster)  [unwired: 1 in]
          }
        }
        n306 = call "RDS Serial Handler Close.vi"("RDS Serial Instrument in"=w729) -> ("error out"=w727:errorcluster, "RDS Serial Instrument out"=w728:refnum<class "RDS Serial Instrument.lvclass">)  [unwired: 9 in]
        n307 = Merge Errors(w727, w724, w723) -> (w722:errorcluster)
      }
    }
    n308 = call "RDS Read Connected.vi"("error in (no error)"=w646, "RDS Serial Instrument in"=w649) -> ("error out"=w647:errorcluster, "Connected"=→"LSR Connected":bool, "RDS Serial Instrument out"=w648:refnum<class "RDS Serial Instrument.lvclass">)  [unwired: 7 in]
  }
  n309 = Unbundle By Name(w5) -> ("device ID"=w4:refnum<k1>)
  n310 = call-poly <vilib>:"Close Input Device.vi"("device ID"=w4) -> ("error out"=w3:errorcluster)  [unwired: 9 in]
  n311 = call <vilib>:"Clear Errors.vi"("error in (no error)"=w3) -> ()  [unwired: 5 in, 2 out]
